vi "AT901 - Queue Steuerung.vi"() -> ()   [LabVIEW 2017]
uses:
  AT901 API/Structures/Struct SystemUnits.ctl
  AT901 API/TypeDefinitions/ES_LengthUnit.ctl
  AT901 API/TypeDefinitions/ES_AngleUnit.ctl
  AT901 API/TypeDefinitions/ES_TemperatureUnit.ctl
  AT901 API/TypeDefinitions/ES_PressureUnit.ctl
  AT901 API/TypeDefinitions/ES_HumidityUnit.ctl
  AT901 API/TypeDefinitions/ES_CoordinateSystemType.ctl
  AT901 API/Structures/Struct EnvironmentData.ctl
  AT901 API/Structures/Struct StationaryModeData.ctl
  AT901 API/TypeDefinitions/ES_ReflectorType.ctl
  AT901 API/Structures/Struct TransformationPoint.ctl
  TypeDefinitions/Queue Steuerung Commands.ctl
  AT901 API/TypeDefinitions/ES_MeasMode.ctl
  AT901 API/Structures/Struct ContinuousTimeModeData.ctl
  AT901 API/TypeDefinitions/ES_RegionType.ctl
  AT901 API/Structures/Struct SystemSettingsData.ctl
  AT901 API/TypeDefinitions/ES_WeatherMonitorStatus.ctl
  AT901 API/Structures/Struct TransformationData.ctl
  <vilib>/Analysis/baseanly.llb/Mean (DBL).vi
  <vilib>/Analysis/NI_AALBase.lvlib
panel:
  in  "Tab Control":T1(tab)
  in  "Connect":bool
  in  "Apply Transformation\nParameters":bool
  in  "Initialize":bool
  in  "GoBirdBath":bool
  in  "GetEnvParams":bool
  out "Environmental Data":T2
  in  "ContMeas":bool
  out "ContMeasResult":dbl[](array[numeric])
  out "Elements in Queue":i32
  in  "SingleMeas":bool
  out "SingleMeasResult":dbl[](array[numeric])
  in  "Punktnummer":string
  in  "Measurement File":path=path "C:/Users/Wehner/Desktop/AT901-MeasFile.txt"
  in  "IP Address":string="192.168.0.1"
  in  "Port":u16=700
  out "XY Graph":cluster{"Array":dbl[], "Array 3":dbl[]}(graph)
  in  "Axis Scaling":dbl(slide) scale=0.0..100.0
  in  "ES ReflectorType":T3=enum."CCR - 1,5 in"
  in  "ES_CoordinateSystemType":T4
  in  "SystemUnits":T5
  in  "Continuous Time Mode Params":T11={"TimeSeparation"=100, "NumberOfPoints"=0}
  in  "StationaryModeData":T12={"Use ADM"=TRUE, "lMeasTime"=500}
  in  "SetPowerLock\nActive":bool=TRUE
  out "Scale":dbl
  in  "Add Actual File":bool
  in  "Add Nominal File":bool
  out "Actual Points Front Indicator":T13(array[cluster])
  in  "Add Actual Point":bool
  in  "Clear Actual":bool
  in  "Remove Actual by Name":bool
  in  "Actual to be Removed":string
  out "Nominal Points Front Indicator":T13(array[cluster])
  in  "Clear Nominal":bool
  in  "Add Nominal":bool
  in  "Remove Nominal by Name":bool
  in  "Nominal to be Removes":string
  in  "CalcTransformation":bool
  out "Translation":dbl[](array[numeric])
  out "Rotation":dbl[](array[numeric])
  out "Nominal Points":T15(array[cluster])
  out "Actual Points":T15(array[cluster])
  # "Single Measurement"
  # "Continuous Measurement"
  # "General Settings"
  # "Continuous Measurement\nSettings"
  # "Single Measurement\nSettings"
  # "Set Nominal Points"
  # "Set Actual Points"
  # "Perform Transformation"
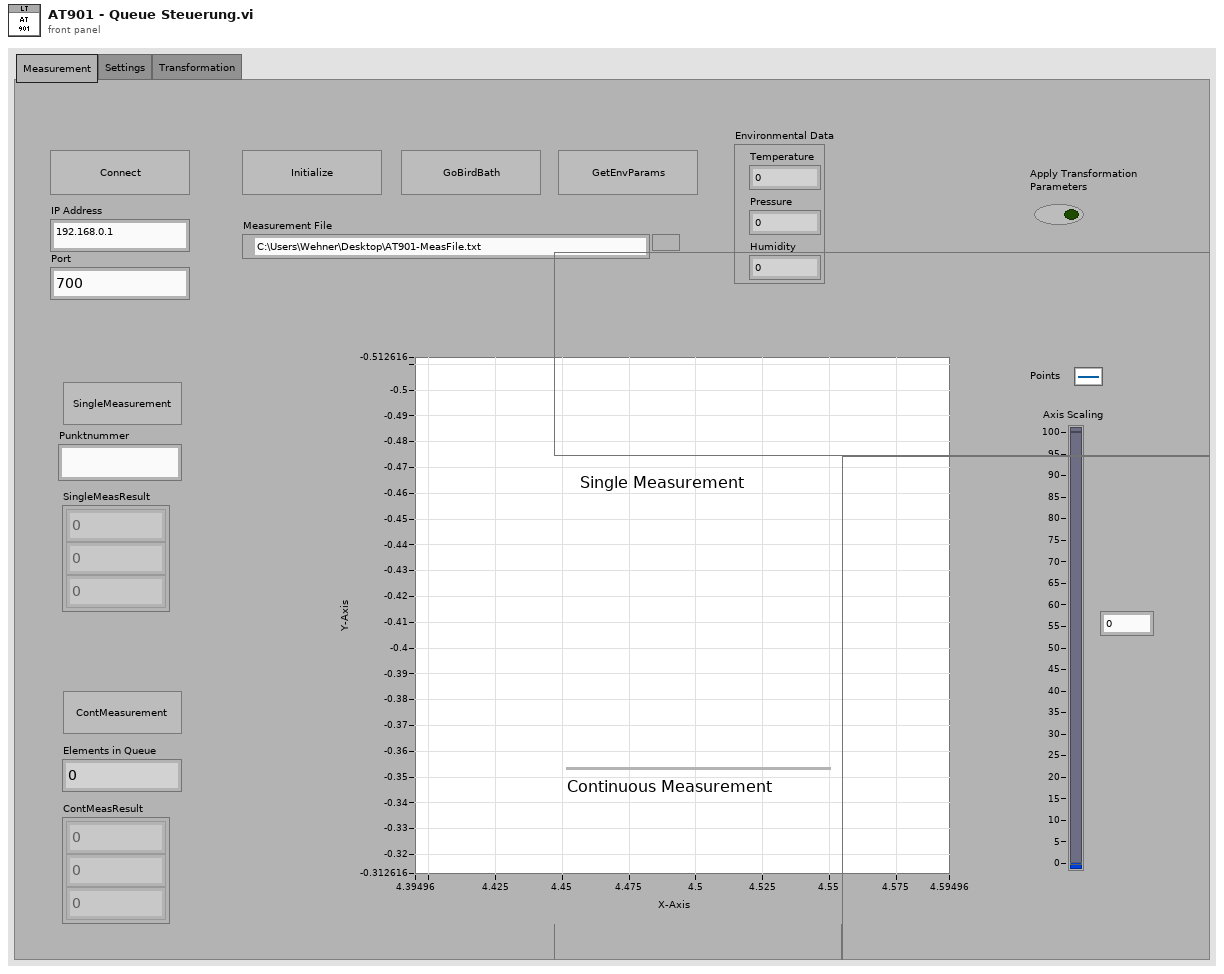
[diagram p1: front panel]
types:
  T1 = enum32{"Measurement", "Settings", "Transformation"}
  T2 = typedef "Struct EnvironmentData.ctl" = cluster{"Temperature":dbl, "Pressure":dbl, "Humidity":dbl}
  T3 = typedef "ES_ReflectorType.ctl" = enum32{"none1", "none2", "CCR - 1,5 in", "none4", "none5", "TBR - 0,5 in", "none7", "CCR - 75mm", "none8", "RRR - 1,5 in"}
  T4 = typedef "ES_CoordinateSystemType.ctl" = enum32{"ES_CS_RHR", "ES_CS_LHRX", "ES_CS_LHRY", "ES_CS_LHRZ", "ES_CS_CCW", "ES_CS_CCC", "ES_CS_SCW", "ES_CS_SCC"}
  T5 = typedef "Struct SystemUnits.ctl" = cluster{"ES_LengthUnit":T6, "ES_AngleUnit":T7, "ES_TemperatureUnit":T8, "ES_PressureUnit":T9, "ES_HumidityUnit":T10}
  T6 = typedef "ES_LengthUnit.ctl" = enum32{"ES_LU__Meter", "ES_LU_Millimeter", "ES_LU_Micron", "ES_LU_Foot", "ES_LU_Yard", "ES_LU_Inch"}
  T7 = typedef "ES_AngleUnit.ctl" = enum32{"ES_AU_Radian", "ES_AU_Degree", "ES_AU_Gon"}
  T8 = typedef "ES_TemperatureUnit.ctl" = enum32{"ES_TU_Celsius", "ES_TU_Fahrenheit"}
  T9 = typedef "ES_PressureUnit.ctl" = enum32{"ES_PU_Mbar", "ES_PU_HPascal", "ES_PU_KPascal", "ES_PU_MmHg", "ES_PU_Psi", "ES_PU_InH2O", "ES_PU_InHg"}
  T10 = typedef "ES_HumidityUnit.ctl" = enum32{"ES_HU_RH"}
  T11 = cluster{"TimeSeparation":u32, "NumberOfPoints":u32}
  T12 = typedef "Struct StationaryModeData.ctl" = cluster{"Use ADM":bool, "lMeasTime":i32}
  T13 = cluster{"X":dbl, "Y":dbl, "Z":dbl, "Punktnummer":string}[]
  T14 = typedef "Struct TransformationPoint.ctl" = cluster{"dVal1":dbl, "dVal2":dbl, "dVal3":dbl, "dStd1":dbl, "dStd2":dbl, "dStd3":dbl, "dCovar12":dbl, "dCovar13":dbl, "dCovar23":dbl}
  T15 = cluster{"Punktnummer":string, "Transformation Point":T14}[]
  T16 = typedef "Queue Steuerung Commands.ctl" = enum16{"Punkte Transformieren", "SetCoordType", "SetStatMeasParams", "AddNominalPoint", "ClearLastActualPoint", "ClearLastNominalPoint", "PowerLock", "AddActualPoint", "CalcTransformation", "SetContTimeParams", "GetEnvParams", "StopContMeas", "GetContMeasData", "StartContMeas", "Idle", "PlotValueChange", "ConnectTracker", "AddNominalPointFile", "AddActualPointFile", "RemoveNominalByName", "RemoveActualByName", "Stop", "Initialise", "SetUnits", "SetReflector", "SingleMeasurement", "GoBirdBath"}
  T17 = typedef "ES_MeasMode.ctl" = enum32{"ES_MM_Stationary", "ES_MM_ContinuousTime", "ES_MM_ContinuousDistance", "ES_MM_Grid", "ES_MM_SphrereCenter", "ES_MM_CircleCenter", "ES_MM_6DStationary", "ES_MM_6DContinuousTime", "ES_MM_6DContinuousDistance", "ES_MM_6DGrid", "ES_MM_6DSphrereCenter", "ES_MM6DCircleCenter"}
  T18 = typedef "Struct ContinuousTimeModeData.ctl" = cluster{"TimeSeparation":u32, "NumberOfPoints":u32, "UseRegion":bool, "ES_RegionType":T19}
  T19 = typedef "ES_RegionType.ctl" = enum32{"ES_RT_Sphere", "ES_RT_Box"}
  T20 = typedef "Struct SystemSettingsData.ctl" = cluster{"WeatherMonitorStatus":T21, "ApplyTransformationParams":bool, "ApplyStationOrientationParams":bool, "KeepLastPosition":bool, "SendUnsolicitedMessages":bool, "SendReflectorPositionData":bool, "TryMeasurementMode":bool, "HasNivel":bool, "HasVideoCamera":bool}
  T21 = typedef "ES_WeatherMonitorStatus.ctl" = enum16{"ES_WMS_NotConnected", "ES_WMS_ReadOnly", "ES_WMS_ReadAndCalculateRefractions"}
  T22 = typedef "Struct TransformationData.ctl" = cluster{"dVal1":dbl, "dVal2":dbl, "dVal3":dbl, "dRot1":dbl, "dRot2":dbl, "dRot3":dbl, "dScale":dbl}
  T23 = typedef "Struct TransformationPointWithPointnumber.ctl" = cluster{"Punktnummer":string, "Transformation Point":T14}
  T24 = typedef "Struct CallTrafo.ctl" = cluster{"dTransVal1":dbl, "dTransVal2":dbl, "dTransVal3":dbl, "dRot1":dbl, "dRot2":dbl, "dRot3":dbl, "dScale":dbl, "dTransVal1 Std":dbl, "dTransVal2 Std":dbl, "dTransVal3 Std":dbl, "dRot1 Std":dbl, "dRot2 Std":dbl, "dRot3 Std":dbl, "dScale Std":dbl, "dRMS":dbl, "dMaxDev":dbl, "dVarianceFactor":dbl}
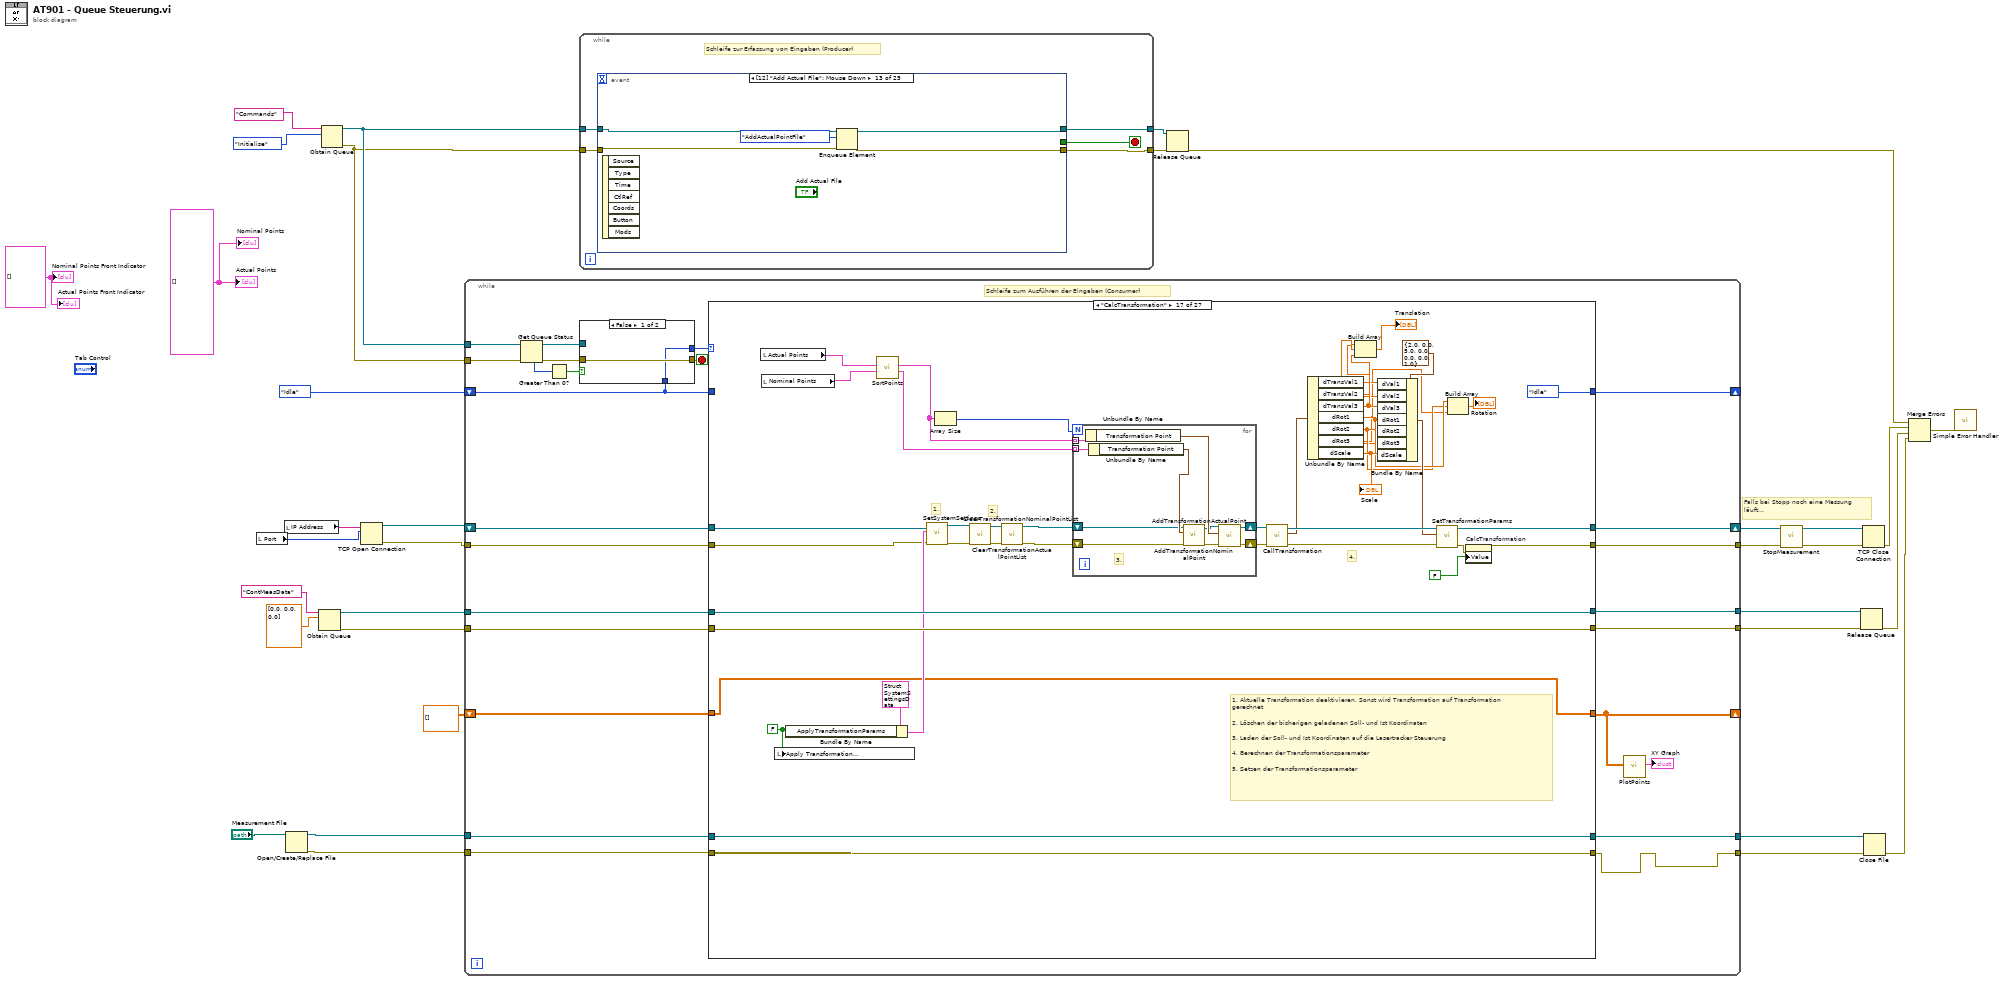
[diagram p0: block diagram]
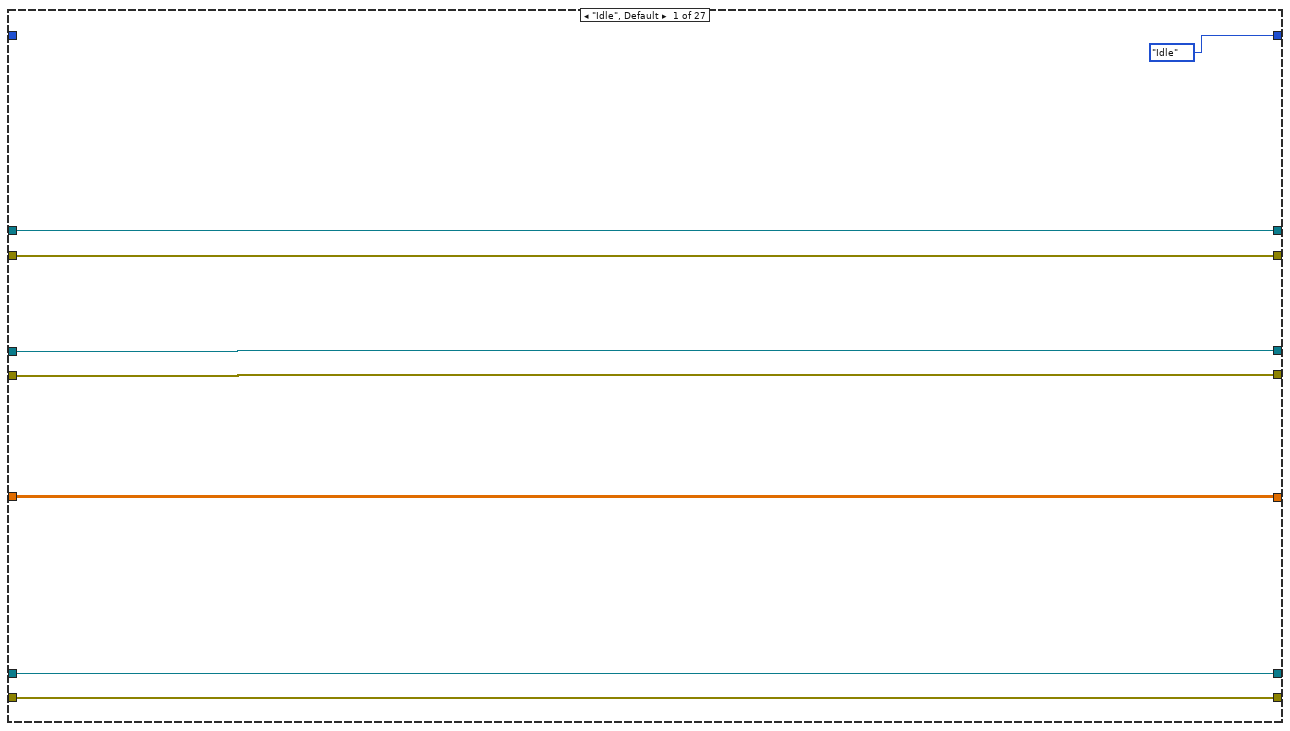
[diagram p2: hidden frame]
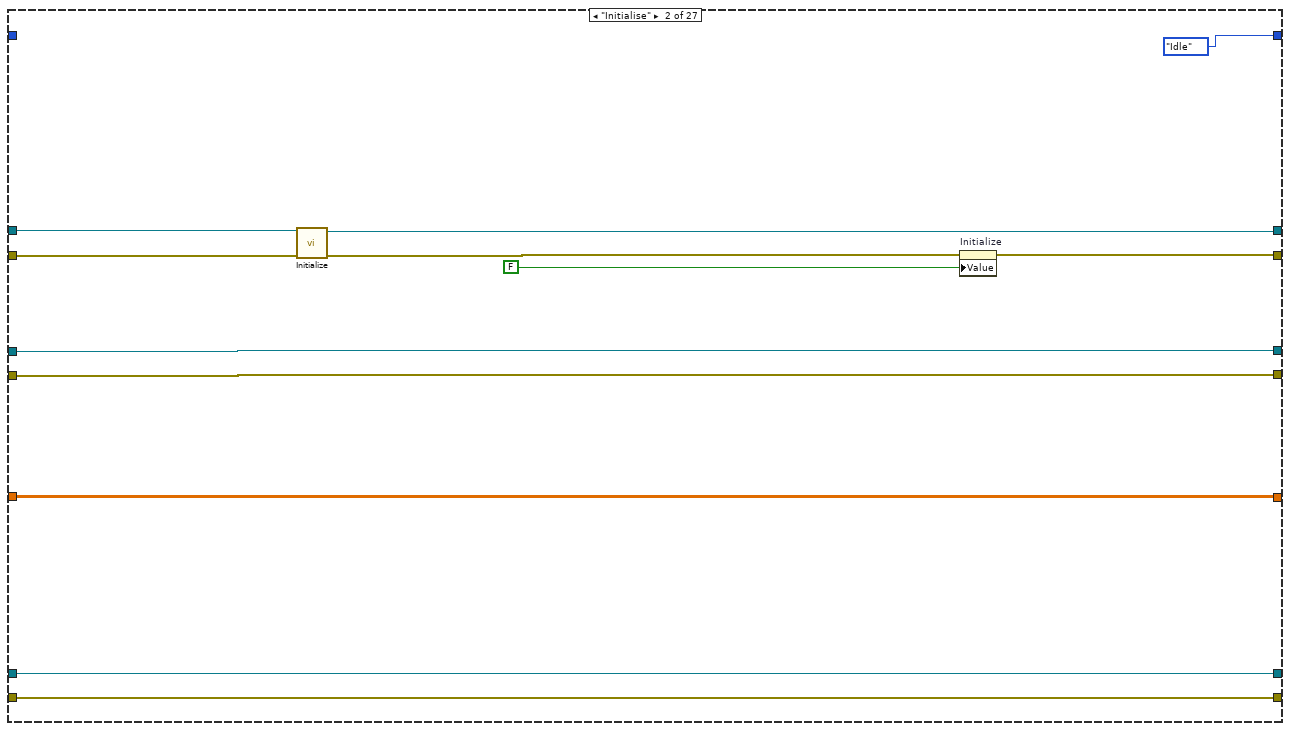
[diagram p3: hidden frame]
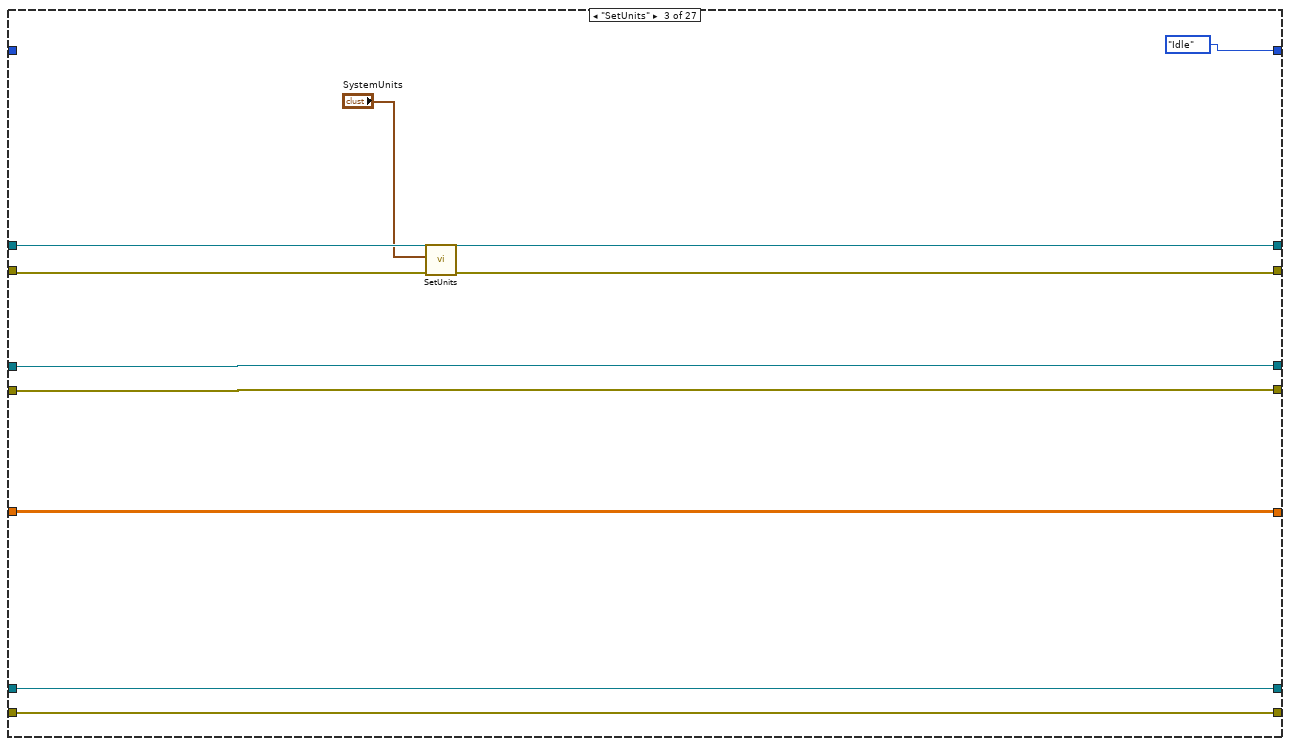
[diagram p4: hidden frame]
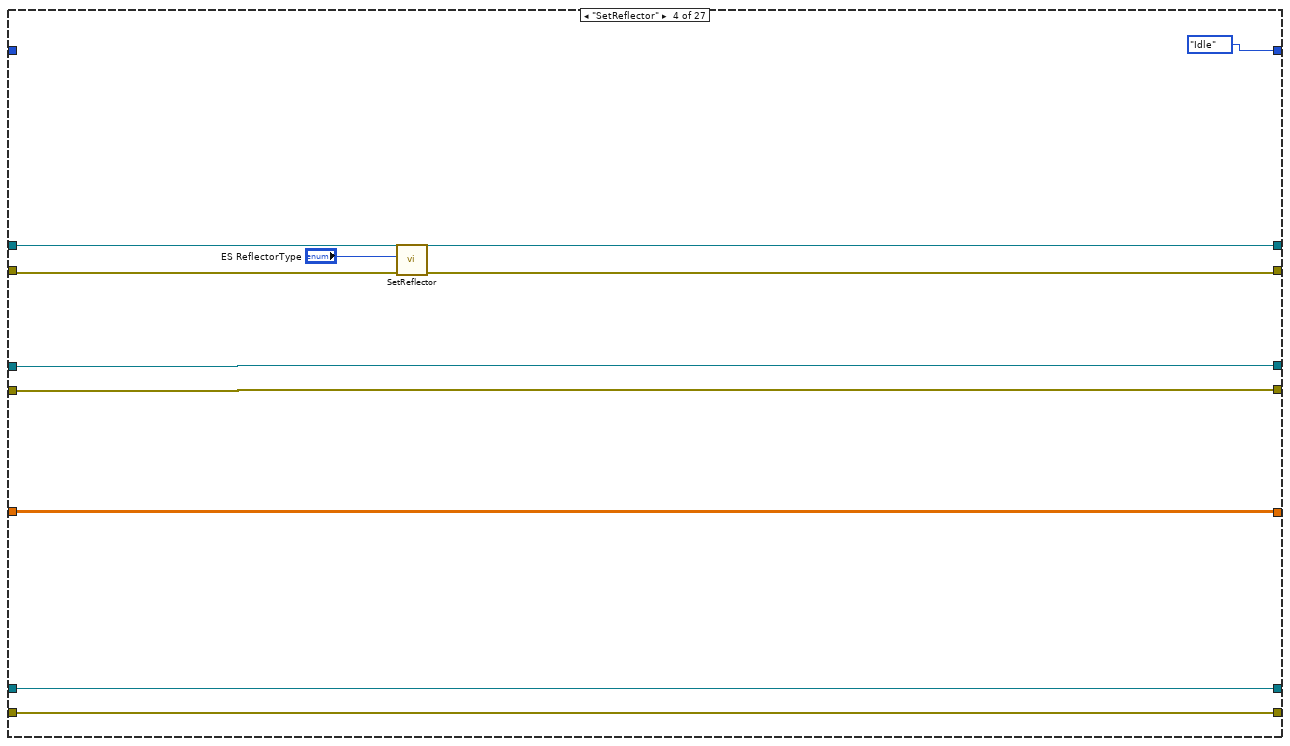
[diagram p5: hidden frame]
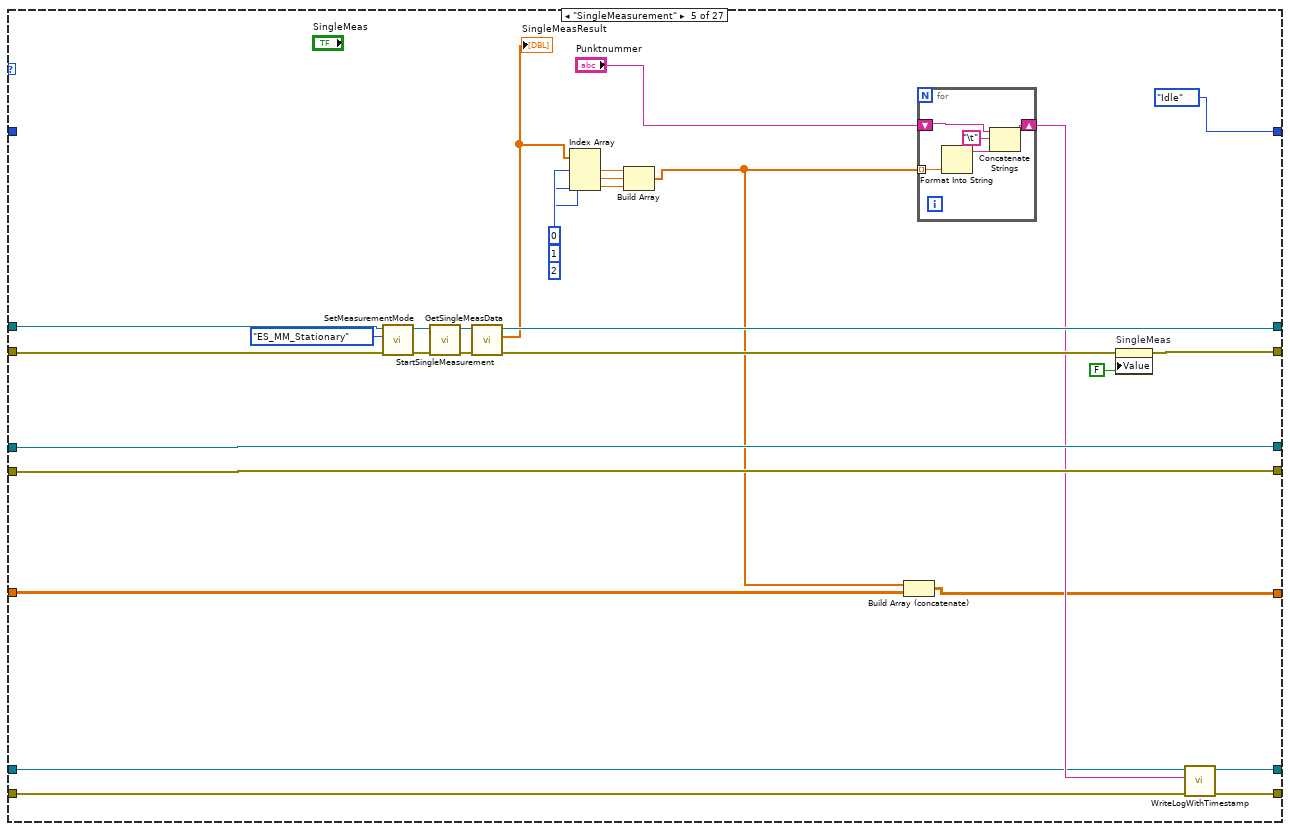
[diagram p6: hidden frame]
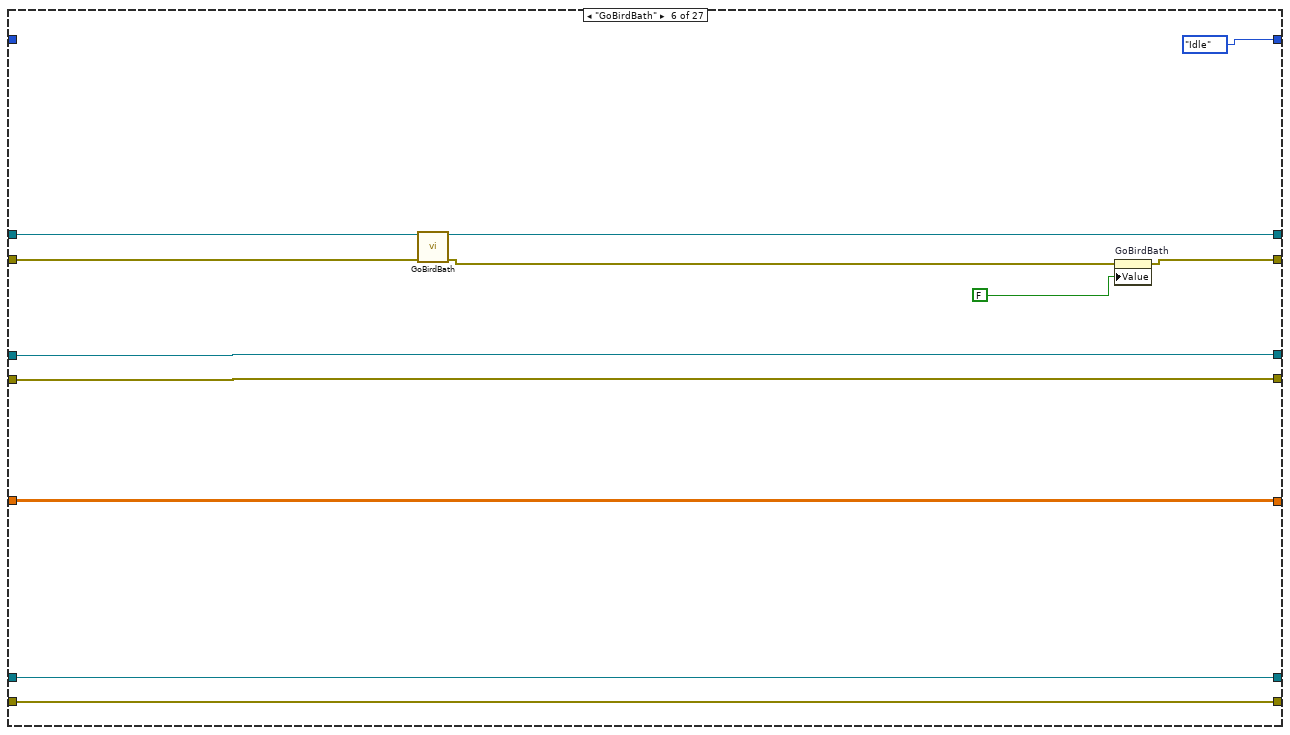
[diagram p7: hidden frame]
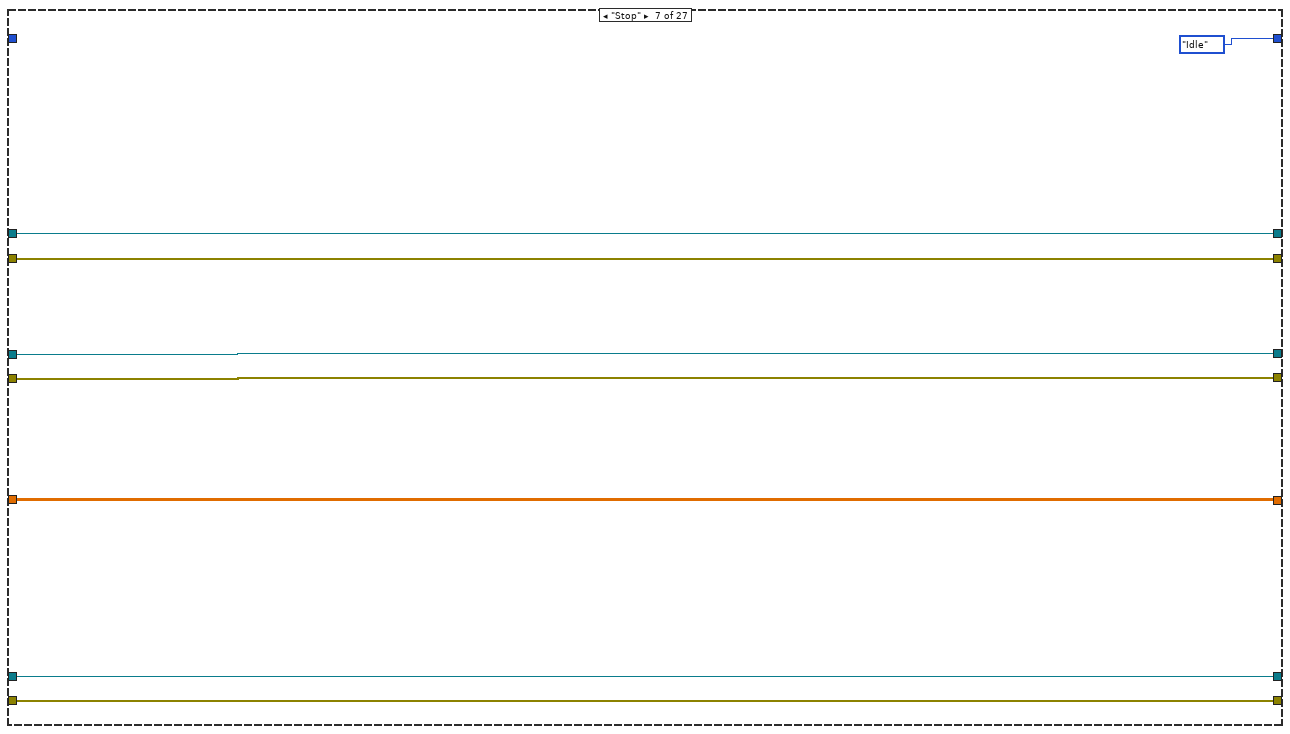
[diagram p8: hidden frame]
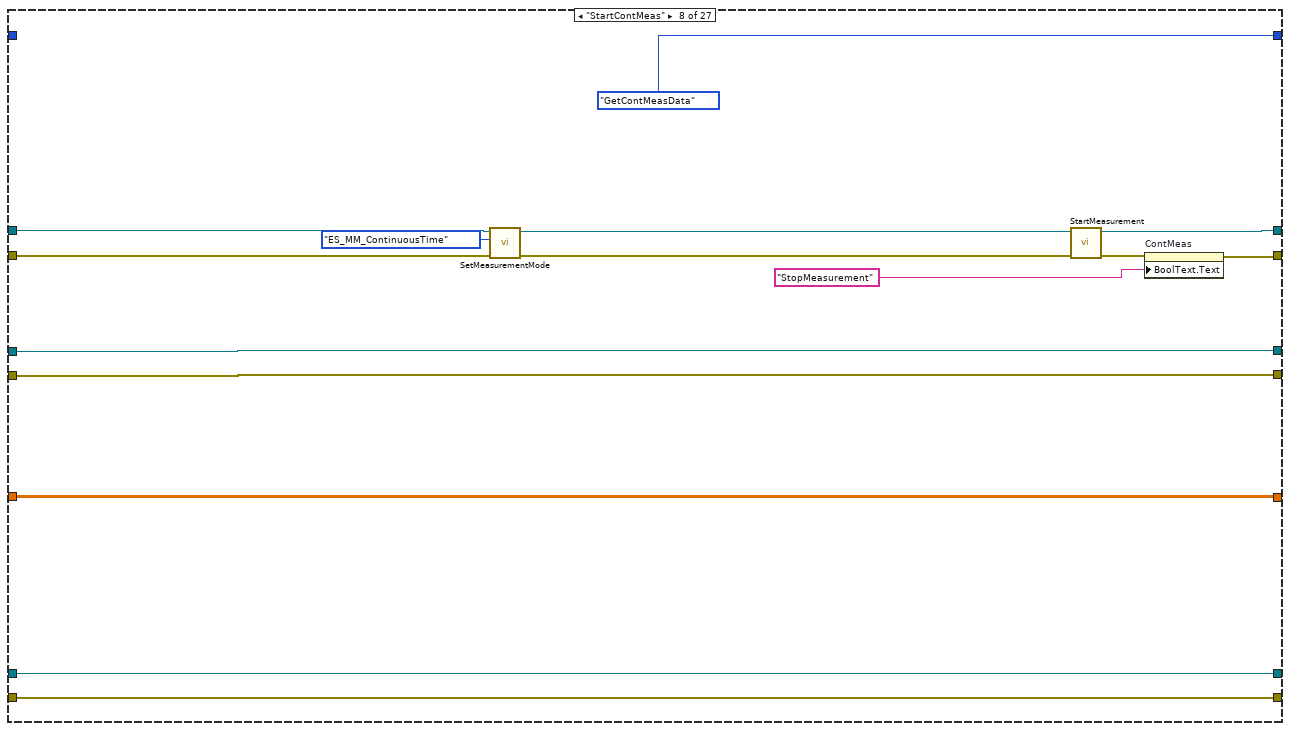
[diagram p9: hidden frame]
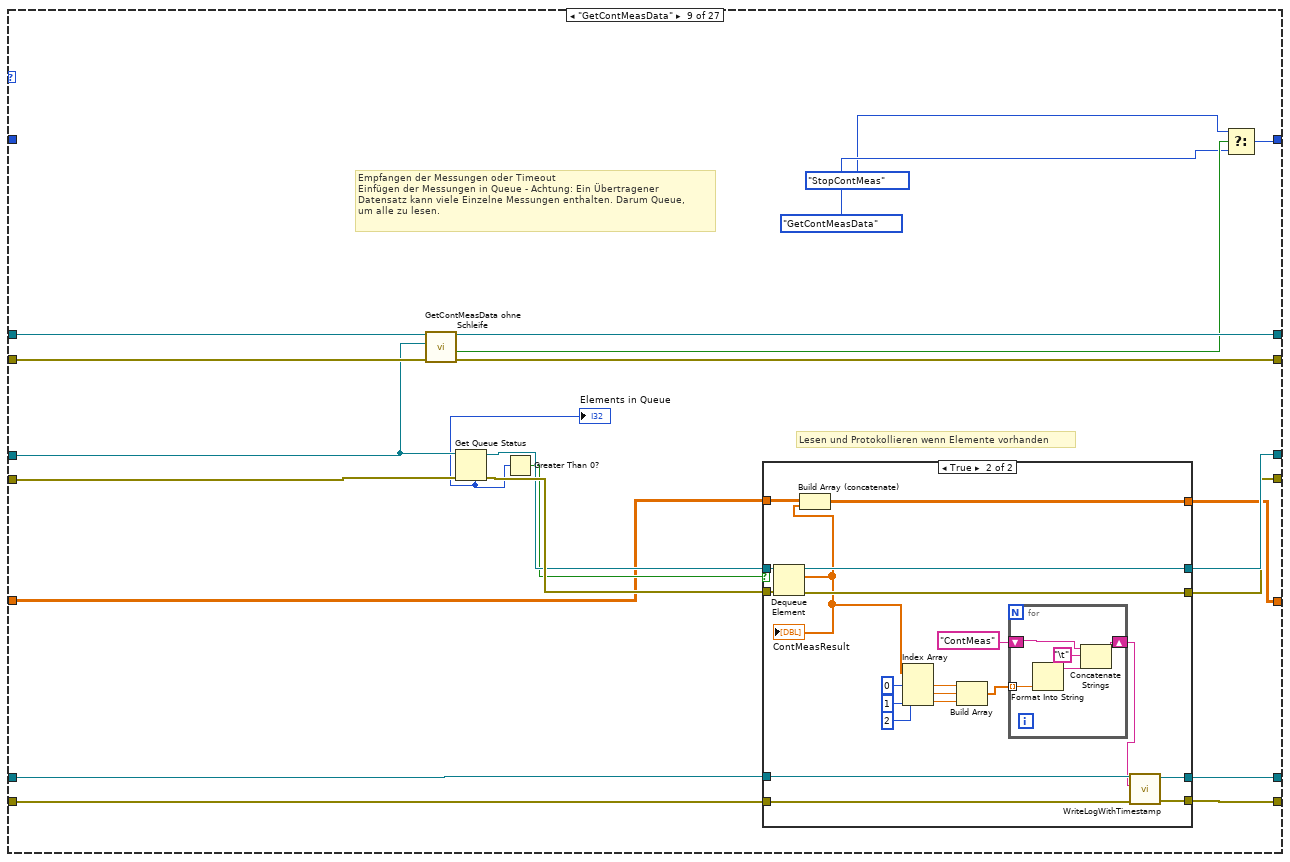
[diagram p10: hidden frame]
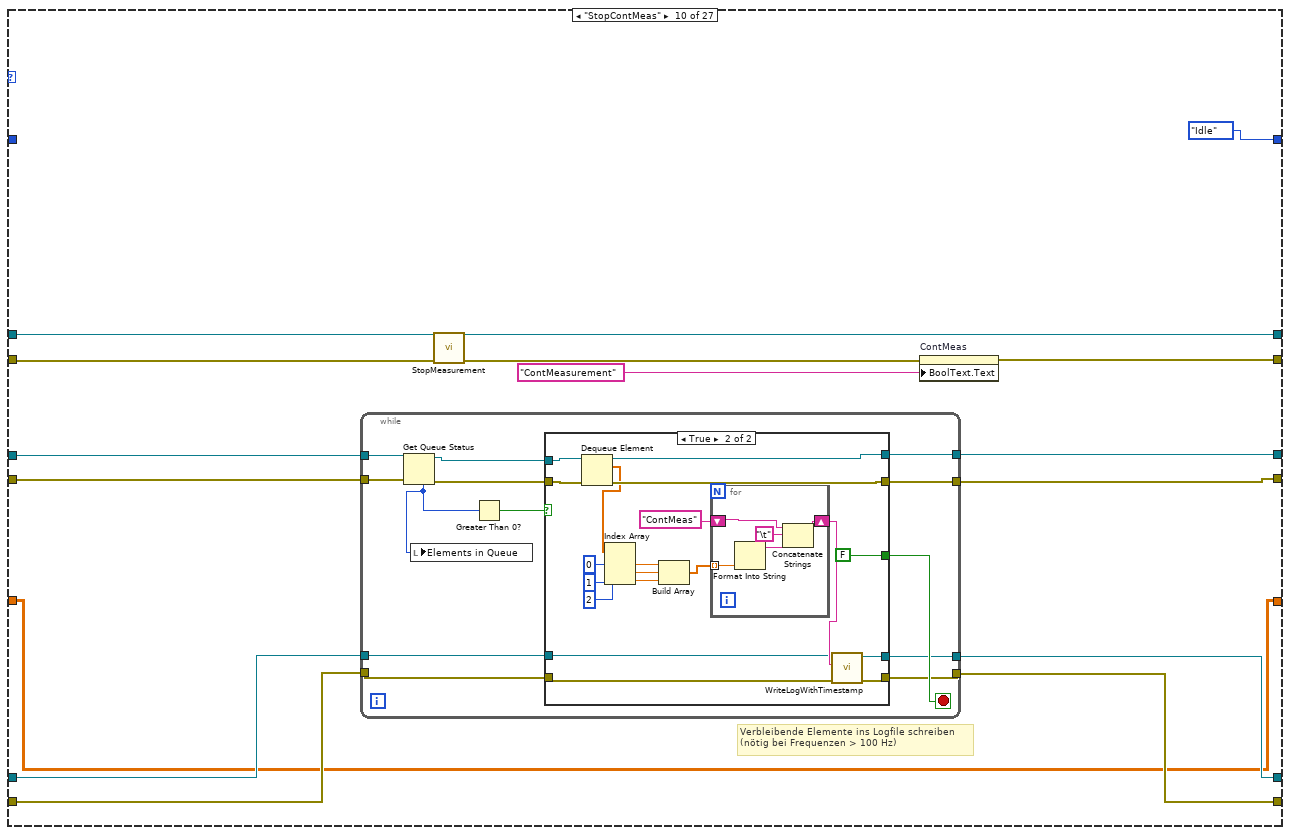
[diagram p12: hidden frame]
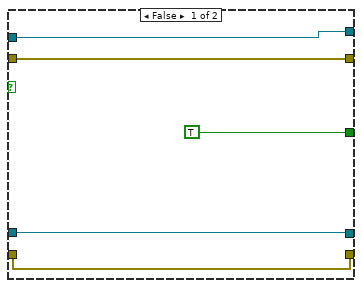
[diagram p13: hidden frame]
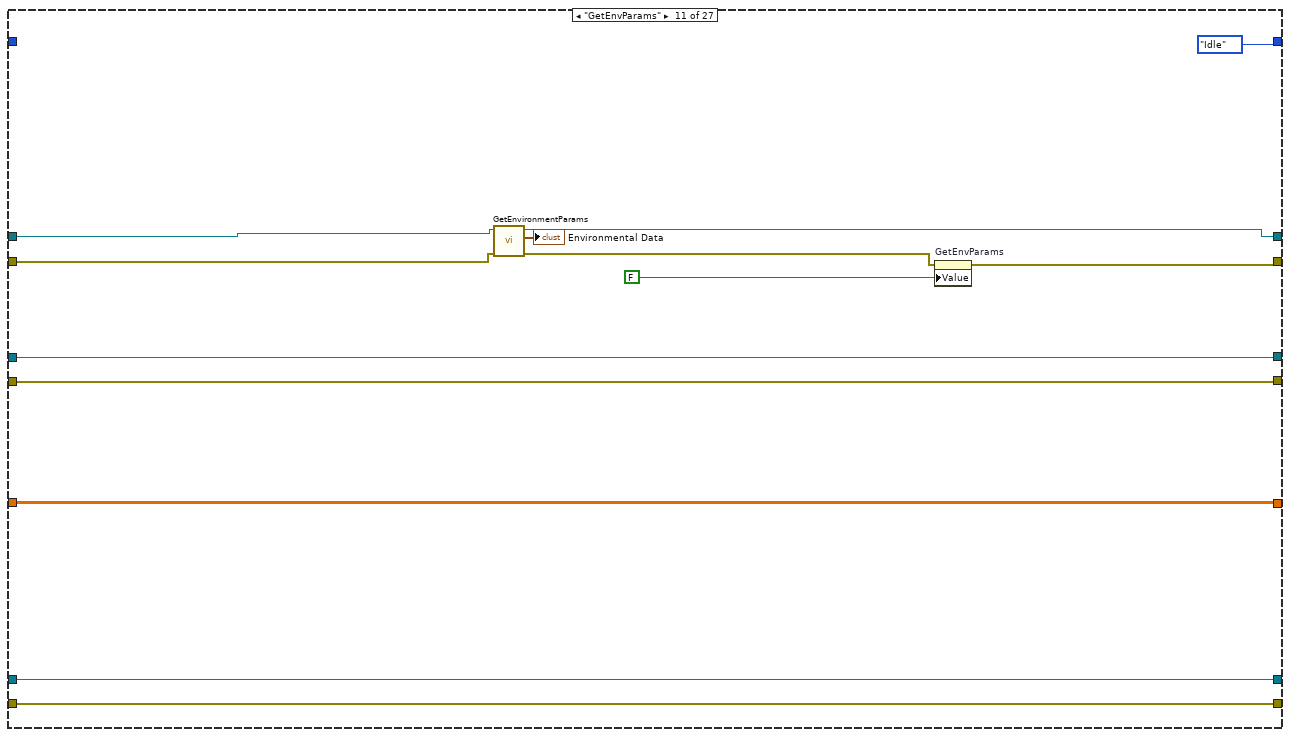
[diagram p14: hidden frame]
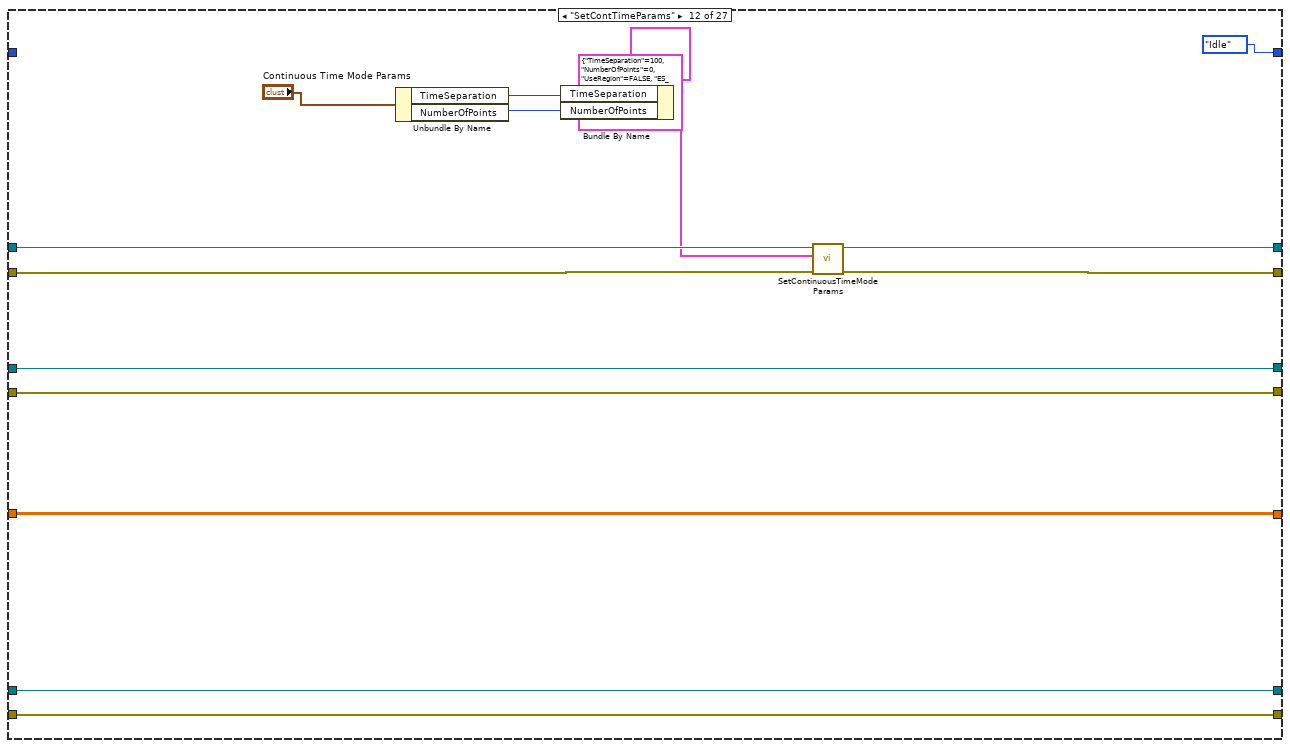
[diagram p15: hidden frame]
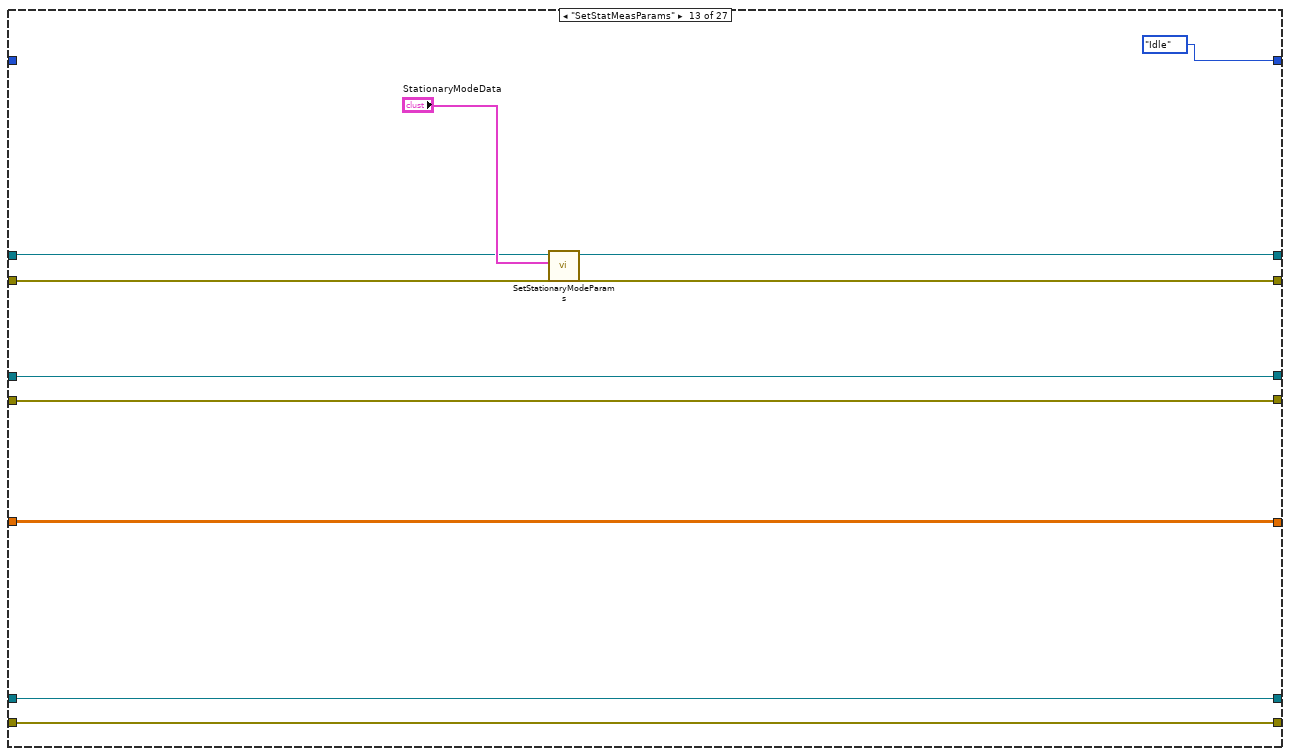
[diagram p16: hidden frame]
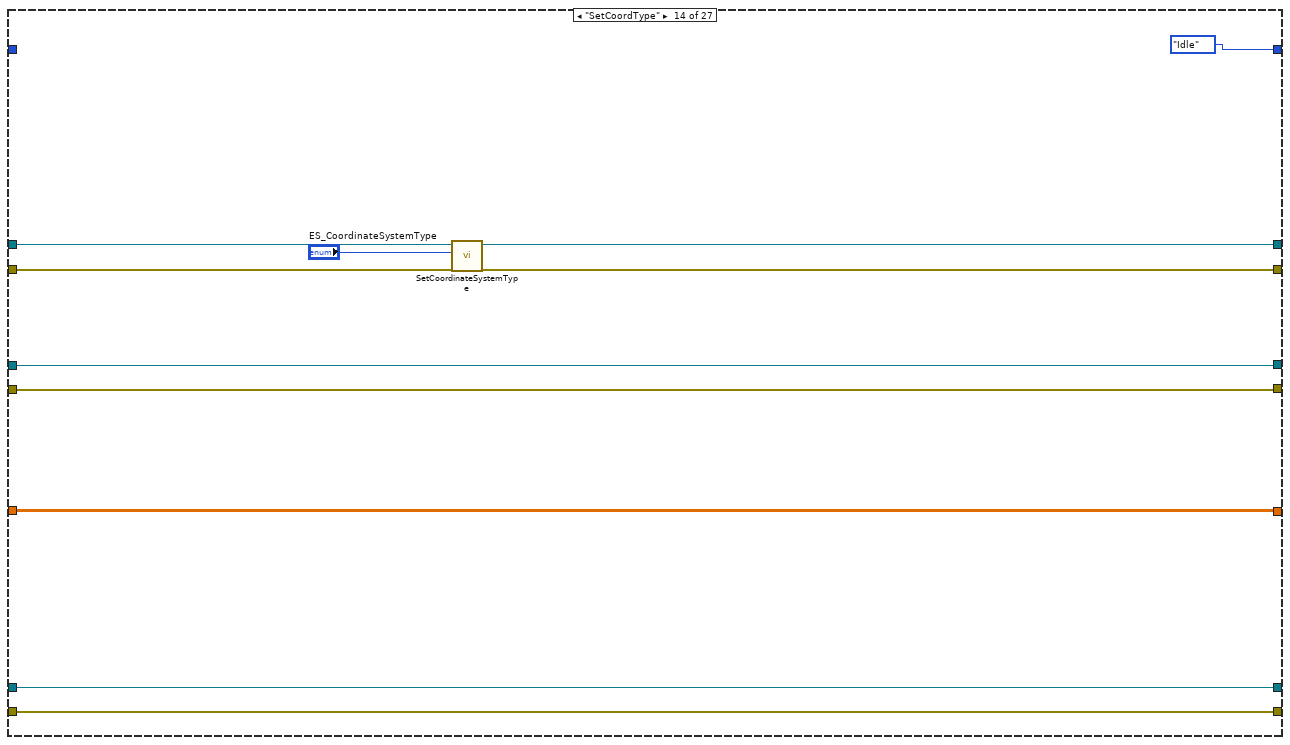
[diagram p17: hidden frame]
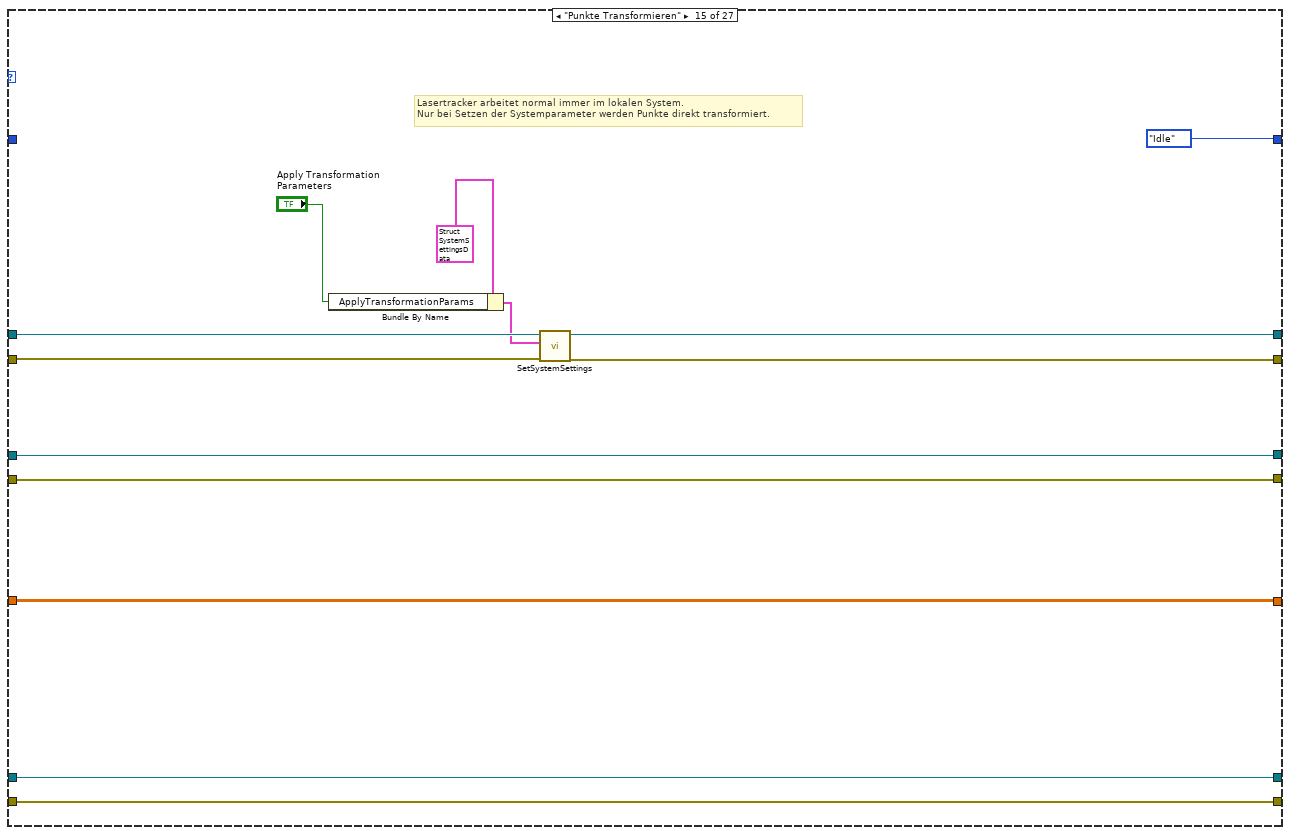
[diagram p18: hidden frame]
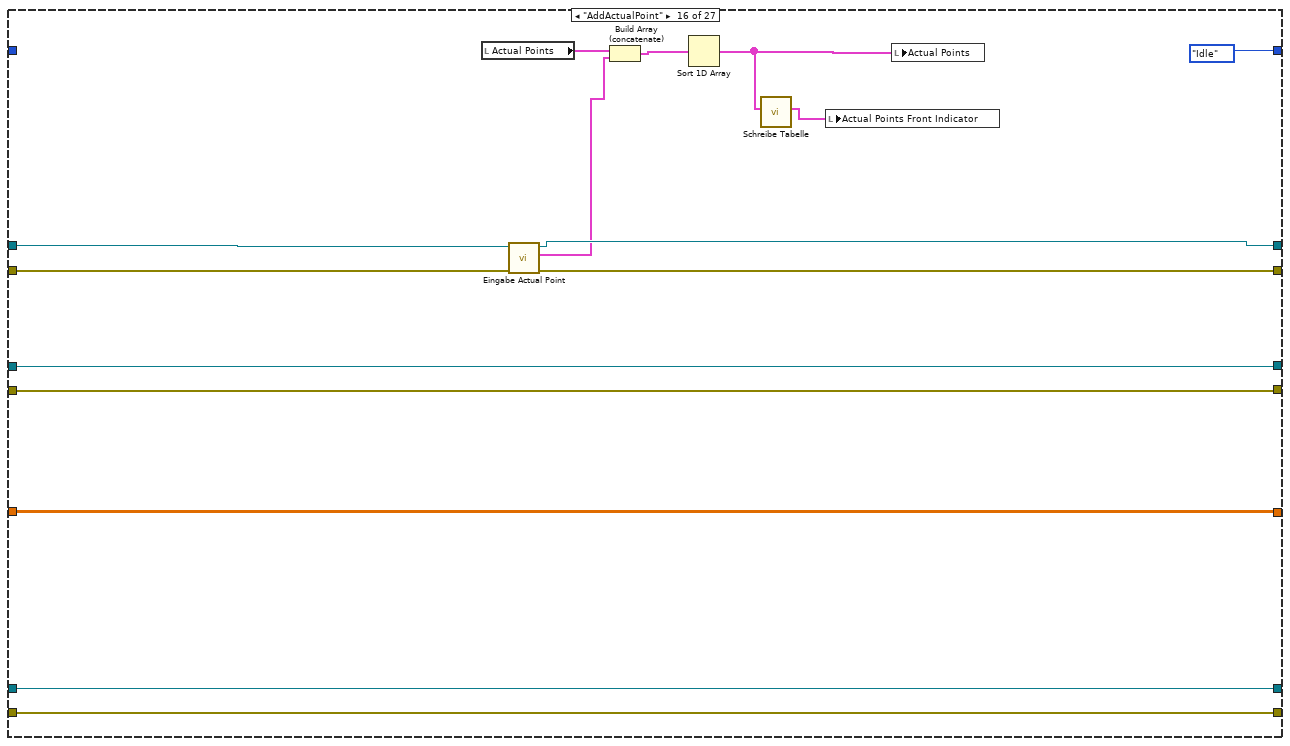
[diagram p19: hidden frame]
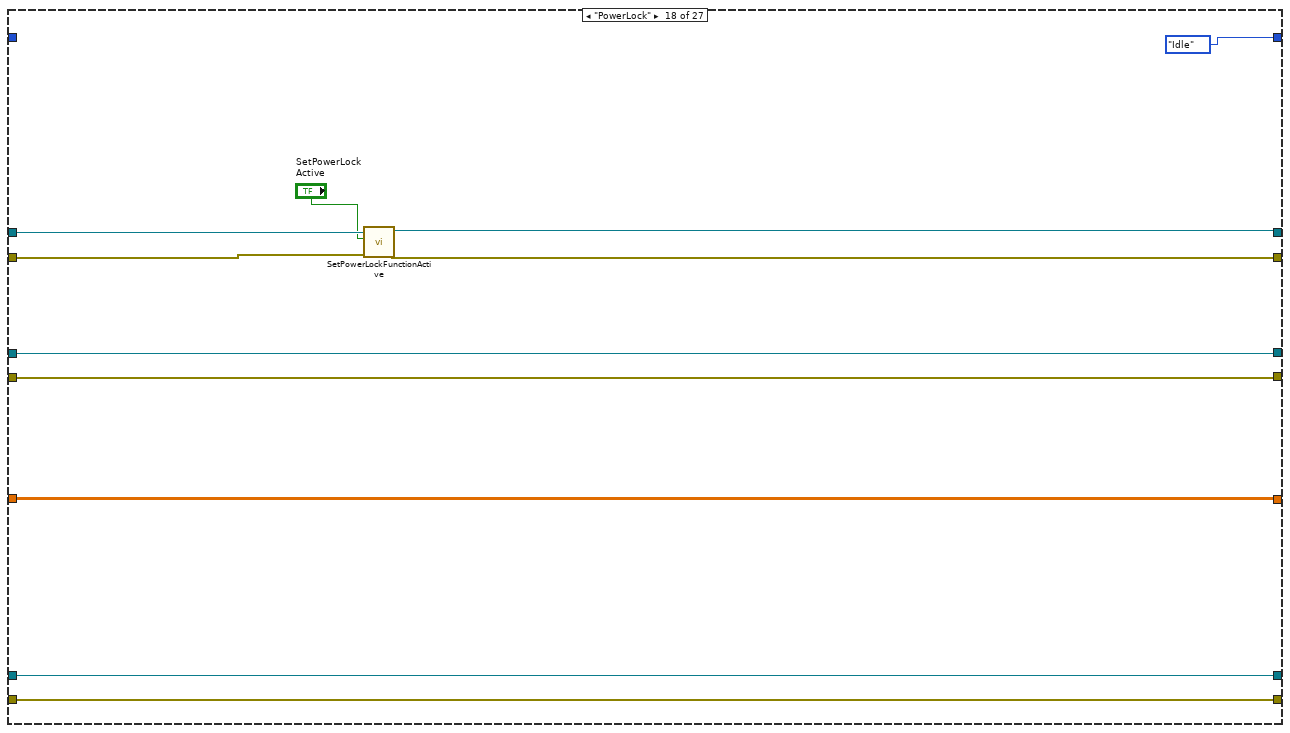
[diagram p20: hidden frame]
diagram:
  w13 = T13 [] ("Nominal Points")
  w14 = T15 [] ("Actual Points")
  # "Falls bei Stopp noch eine Messung\nläuft..."
  n1 = local read "Port"() -> (w4:u16)
  n2 = local read "IP Address"() -> (w5:string)
  n3 = Open/Create/Replace File(file path (use dialog)="Measurement File") -> (refnum out=w18:refnum<file>, error out=w2:errorcluster)  [unwired: 5 in, 1 out]
  n4 = Obtain Queue(name (unnamed)="ContMeasData", element data type=dbl[] [0.0, 0.0, 0.0] ("Meas Result")) -> (queue out=w25:refnum<queue>, error out=w24:errorcluster)  [unwired: 3 in, 1 out]
  n5 = Obtain Queue(name (unnamed)="Commands", element data type=Queue_Steuerung_Commands."Initialise") -> (queue out=w30:refnum<queue>, error out=w29:errorcluster)  [unwired: 3 in, 1 out]
  n6 = TCP Open Connection(address=w5, remote port or service name=w4) -> (connection ID=w7:refnum<k5>, error out=w6:errorcluster)  [unwired: 3 in]
  n7 = while {
    tunnel: w30 -> [w59]
    tunnel: w6 -> [w51]
    tunnel: [w50] -> w11
    tunnel: w29 -> [w49]
    shift-right: [w47] -> _
    shift-left: Queue_Steuerung_Commands."Idle" -> [w35]
    tunnel: w25 -> [w46]
    tunnel: w24 -> [w45]
    tunnel: [w44] -> w23
    tunnel: [w43] -> w22
    tunnel: w18 -> [w40]
    tunnel: w2 -> [w41]
    tunnel: [w42] -> w17
    shift-right: [w53] -> w8
    shift-left: w7 -> [w52]
    shift-right: [w38] -> _
    shift-left: dbl[][] [] -> [w39]
    tunnel: [w36] -> w1
    stop <- w48 stop-if-true
    # "Schleife zum Ausführen der Eingaben (Consumer)"
    n8 = Get Queue Status(queue=w59, error in (no error)=w49) -> (queue out=w57:refnum<queue>, error out=w56:errorcluster, # elements in queue=w58:i32)  [unwired: 1 in, 5 out]
    n9 = Greater Than 0?(x=w58) -> (x > 0?=w55:bool)
    n10 = case shown="False" w55 {
      tunnel: w57 -> [_ w558]
      tunnel: w56 -> [w554 w557]
      tunnel: [w553 w556] -> w54
      tunnel: [w554 w555] -> w48
      tunnel: w35 -> [w553 _]
      frame False {
      }
      frame True {
        n11 = Dequeue Element(queue=w558, error in (no error)=w557) -> (element=w556:T16, error out=w555:errorcluster)  [unwired: 1 in, 2 out]
      }
    }
    n12 = case shown="\"CalcTransformation\"" w54 {
      tunnel: [w67 w77 w85 w96 w126 w143 w156 w166 w190 w237 w290 w305 w315 w326 w338 w354 w391 w415 w435 w449 w463 w477 w491 w505 w519 w526 w552] -> w53
      tunnel: w52 -> [w67 w79 w88 w99 w129 w148 w156 w168 w193 w239 w292 w306 w317 w329 w340 w355 w382 w418 w435 w449 w463 w477 w491 w505 w519 _ w552]
      tunnel: w51 -> [w66 w78 w87 w98 w125 w147 w155 w167 w192 w238 w291 w307 w316 w328 w339 w352 w383 w417 w434 w448 w462 w467 w481 w494 w511 w525 w547]
      tunnel: [w66 w75 w86 w97 w121 w144 w155 w161 w191 w235 w286 w304 w314 w327 w337 w353 w376 w414 w434 w448 w462 w466 w482 w493 w510 w522 w546] -> w50
      tunnel: [Queue_Steuerung_Commands."Idle" Queue_Steuerung_Commands."Idle" Queue_Steuerung_Commands."Idle" Queue_Steuerung_Commands."Idle" Queue_Steuerung_Commands."Idle" Queue_Steuerung_Commands."Idle" Queue_Steuerung_Commands."Idle" Queue_Steuerung_Commands."GetContMeasData" w186 Queue_Steuerung_Commands."Idle" Queue_Steuerung_Commands."Idle" Queue_Steuerung_Commands."Idle" Queue_Steuerung_Commands."Idle" Queue_Steuerung_Commands."Idle" Queue_Steuerung_Commands."Idle" Queue_Steuerung_Commands."Idle" Queue_Steuerung_Commands."Idle" Queue_Steuerung_Commands."Idle" Queue_Steuerung_Commands."Idle" Queue_Steuerung_Commands."Idle" Queue_Steuerung_Commands."Idle" Queue_Steuerung_Commands."Idle" Queue_Steuerung_Commands."Idle" Queue_Steuerung_Commands."Idle" Queue_Steuerung_Commands."Idle" Queue_Steuerung_Commands."Idle" w534] -> w47
      tunnel: w46 -> [w65 w73 w90 w101 w120 w142 w154 w164 w183 w233 w294 w309 w320 w331 w344 w359 w401 w422 w433 w447 w461 w476 w490 w504 w518 w532 w551]
      tunnel: w45 -> [w64 w72 w89 w100 w119 w141 w153 w163 w182 w232 w293 w308 w319 w330 w343 w358 w400 w421 w432 w446 w460 w475 w489 w503 w517 w531 w550]
      tunnel: [w65 w73 w90 w101 w120 w142 w154 w164 w181 w230 w294 w309 w320 w331 w344 w359 w401 w422 w433 w447 w461 w476 w490 w504 w518 w532 w551] -> w44
      tunnel: [w64 w72 w89 w100 w119 w141 w153 w163 w180 w231 w293 w308 w319 w330 w343 w358 w400 w421 w432 w446 w460 w475 w489 w503 w517 w531 w550] -> w43
      tunnel: w41 -> [w63 w71 w83 w94 w106 w140 w152 w159 w175 w228 w285 w303 w313 w324 w342 w357 w399 w420 w431 w445 w459 w474 w488 w502 w516 w530 w549]
      tunnel: w40 -> [w62 w70 w82 w93 w107 w139 w151 w158 w174 w229 w284 w302 w312 w323 w341 w356 w398 w419 w430 w444 w458 w473 w487 w501 w515 w529 w548]
      tunnel: [w63 w71 w83 w94 w118 w140 w152 w159 w176 w227 w285 w303 w313 w324 w342 w357 w399 w420 w431 w445 w459 w474 w488 w502 w516 w530 w549] -> w36
      tunnel: [w62 w70 w82 w93 w117 w139 w151 w158 w177 w226 w284 w302 w312 w323 w341 w356 w398 w419 w430 w444 w458 w473 w487 w501 w515 w529 w548] -> w42
      tunnel: [w60 w68 w80 w91 w103 w137 w149 w157 w172 w224 w282 w295 w310 w321 w332 w345 w369 w412 w423 w436 w450 w464 w478 w492 w506 w520 w544] -> w38
      tunnel: w39 -> [w60 w68 w80 w91 w102 w137 w149 w157 w173 w224 w282 w295 w310 w321 w332 w345 w369 w412 w423 w436 w450 w464 w478 w492 w506 w520 w544]
      tunnel: w35 -> [_ _ _ _ _ _ _ _ _ _ _ _ _ _ _ _ _ _ _ _ _ _ _ _ _ _ w534]
      frame "Idle", Default {
      }
      frame "Initialise" {
        n13 = call "Initialize.vi"("error in (no error)"=w78, "TCP Network Connection in"=w79) -> ("error out"=w76:errorcluster, "TCP Network Connection out"=w77:refnum<k5>)  [unwired: 6 in, 2 out]
        n14 = property on="Initialize" class="Bool (strict)"(error in=w76, "Value"=FALSE ("Initialize")) -> (error out=w75:errorcluster)  [unwired: 1 in, 1 out]
      }
      frame "SetUnits" {
        n15 = call "SetUnits.vi"("error in (no error)"=w87, "SystemUnits"="SystemUnits", "TCP Network Connection in"=w88) -> ("error out"=w86:errorcluster, "TCP Network Connection out"=w85:refnum<k5>)  [unwired: 5 in, 2 out]
      }
      frame "SetReflector" {
        n16 = call "SetReflector.vi"("error in (no error)"=w98, "ES ReflectorType"="ES ReflectorType", "TCP Network Connection in"=w99) -> ("error out"=w97:errorcluster, "TCP Network Connection out"=w96:refnum<k5>)  [unwired: 5 in, 2 out]
      }
      frame "SingleMeasurement" {
        n17 = call "SetMeasurementMode.vi"("error in (no error)"=w125, "ES_MeasMode"=ES_MeasMode."ES_MM_Stationary", "TCP Network Connection in"=w129) -> ("error out"=w130:errorcluster, "TCP Network Connection out"=w128:refnum<k5>)  [unwired: 5 in, 2 out]
        n18 = call "StartSingleMeasurement.vi"("error in (no error)"=w130, "TCP Network Connection in"=w128) -> ("error out"=w131:errorcluster, "TCP Network Connection out"=w127:refnum<k5>)  [unwired: 7 in, 1 out]
        n19 = call "GetSingleMeasData.vi"("error in (no error)"=w131, "TCP Network Connection in"=w127) -> ("error out"=w122:errorcluster, "Meas Result"=w113:dbl[], "TCP Network Connection out"=w126:refnum<k5>)  [unwired: 6 in, 1 out]
        "SingleMeasResult" <- w113
        n20 = Index Array(array=w113, index #1=0 ("index"), index #2=1 ("index"), index #3=2 ("index")) -> (element #1=w112:dbl, element #2=w111:dbl, element #3=w110:dbl)
        n21 = Build Array(w112, w111, w110) -> (w104:dbl[])
        n22 = Build Array (concatenate)(w104, w102) -> (w103:dbl[][])
        n23 = for {
          tunnel: w104 -> [w136] mode=indexing
          shift-right: [w133] -> w108
          shift-left: "Punktnummer" -> [w134]
          n24 = Format Into String(w136) -> (resulting string=w135:string)  [unwired: 3 in, 1 out]
          n25 = Concatenate Strings(w134, "\t", w135) -> (w133:string)
        }
        n26 = property on="SingleMeas" class="Bool (strict)"(error in=w122, "Value"=FALSE ("SingleMeas")) -> (error out=w121:errorcluster)  [unwired: 1 in, 1 out]
        n27 = call "WriteLogWithTimestamp.vi"("error in (no error)"=w106, "Punktnummer"=w108, "Byte Stream File in"=w107) -> ("error out"=w118:errorcluster, "Byte Stream File out"=w117:refnum<file>)  [unwired: 7 in]
      }
      frame "GoBirdBath" {
        n28 = call "GoBirdBath.vi"("error in (no error)"=w147, "TCP Network Connection in"=w148) -> ("error out"=w145:errorcluster, "TCP Network Connection out"=w143:refnum<k5>)  [unwired: 6 in, 2 out]
        n29 = property on="GoBirdBath" class="Bool (strict)"(error in=w145, "Value"=FALSE ("GoBirdBath")) -> (error out=w144:errorcluster)  [unwired: 1 in, 1 out]
      }
      frame "Stop" {
      }
      frame "StartContMeas" {
        n30 = call "SetMeasurementMode.vi"("error in (no error)"=w167, "ES_MeasMode"=ES_MeasMode."ES_MM_ContinuousTime", "TCP Network Connection in"=w168) -> ("error out"=w170:errorcluster, "TCP Network Connection out"=w169:refnum<k5>)  [unwired: 5 in, 2 out]
        n31 = call "StartMeasurement.vi"("error in (no error)"=w170, "TCP Network Connection in"=w169) -> ("error out"=w162:errorcluster, "TCP Network Connection out"=w166:refnum<k5>)  [unwired: 6 in, 2 out]
        n32 = property on="ContMeas" class="Bool (strict)"(error in=w162, "BoolText.Text"="StopMeasurement" ("Boolean Text.Text")) -> (error out=w161:errorcluster)  [unwired: 1 in, 1 out]
      }
      frame "GetContMeasData" {
        # "Lesen und Protokollieren wenn Elemente vorhanden"
        # "Empfangen der Messungen oder Timeout\nEinfügen der Messungen in Queue - Achtung: Ein Übertragener\nDatensatz kann viele Einzelne Messungen enthalten. Darum Queue, \num alle zu lesen."
        n33 = call "GetContMeasData ohne Schleife.vi"("error in (no error)"=w192, "queue out"=w183, "TCP Network Connection in"=w193) -> ("error out"=w191:errorcluster, "Messabbruch"=w189:bool, "TCP Network Connection out"=w190:refnum<k5>)  [unwired: 4 in, 2 out]
        n34 = Get Queue Status(queue=w183, error in (no error)=w182) -> (queue out=w184:refnum<queue>, error out=w185:errorcluster, # elements in queue=w178:i32)  [unwired: 1 in, 5 out]
        "Elements in Queue" <- w178
        n35 = Greater Than 0?(x=w178) -> (x > 0?=w179:bool)
        n36 = case shown="True" w179 {
          tunnel: w185 -> [w197 w218]
          tunnel: w184 -> [w198 w217]
          tunnel: [w198 w216] -> w181
          tunnel: [w197 w215] -> w180
          tunnel: [w196 w214] -> w177
          tunnel: [w195 w213] -> w176
          tunnel: w175 -> [w195 w212]
          tunnel: w174 -> [w196 w211]
          tunnel: w173 -> [w194 w201]
          tunnel: [w194 w199] -> w172
          frame False {
          }
          frame True {
            n37 = Dequeue Element(queue=w217, error in (no error)=w218) -> (queue out=w216:refnum<queue>, element=w200:dbl[], error out=w215:errorcluster)  [unwired: 1 in, 1 out]
            "ContMeasResult" <- w200
            n38 = Build Array (concatenate)(w201, w200) -> (w199:dbl[][])
            n39 = Index Array(array=w200, index #1=0 ("index"), index #2=1 ("index"), index #3=2 ("index")) -> (element #1=w207:dbl, element #2=w206:dbl, element #3=w205:dbl)
            n40 = Build Array(w207, w206, w205) -> (w204:dbl[])
            n41 = for {
              tunnel: w204 -> [w223] mode=indexing
              shift-right: [w220] -> w203
              shift-left: "ContMeas" -> [w221]
              n42 = Format Into String(w223) -> (resulting string=w222:string)  [unwired: 3 in, 1 out]
              n43 = Concatenate Strings(w221, "\t", w222) -> (w220:string)
            }
            n44 = call "WriteLogWithTimestamp.vi"("error in (no error)"=w212, "Punktnummer"=w203, "Byte Stream File in"=w211) -> ("error out"=w213:errorcluster, "Byte Stream File out"=w214:refnum<file>)  [unwired: 7 in]
          }
        }
        n45 = Select(t=Queue_Steuerung_Commands."StopContMeas", s=w189, f=Queue_Steuerung_Commands."GetContMeasData") -> (s? t:f=w186:T16)
      }
      frame "StopContMeas" {
        # "Verbleibende Elemente ins Logfile schreiben\n(nötig bei Frequenzen > 100 Hz)"
        n46 = while {
          tunnel: w233 -> [w252]
          tunnel: w232 -> [w251]
          tunnel: [w248] -> w231
          tunnel: [w245] -> w230
          tunnel: w229 -> [w244]
          tunnel: w228 -> [w243]
          tunnel: [w242] -> w227
          tunnel: [w241] -> w226
          stop <- w249 stop-if-true
          n47 = Get Queue Status(queue=w252, error in (no error)=w251) -> (queue out=w246:refnum<queue>, error out=w247:errorcluster, # elements in queue=w240:i32)  [unwired: 1 in, 5 out]
          n48 = local write "Elements in Queue"(w240) -> ()
          n49 = Greater Than 0?(x=w240) -> (x > 0?=w250:bool)
          n50 = case shown="True" w250 {
            tunnel: [TRUE FALSE] -> w249
            tunnel: [w256 w274] -> w248
            tunnel: w247 -> [w256 w272]
            tunnel: w246 -> [w255 w273]
            tunnel: [w255 w275] -> w245
            tunnel: w244 -> [w254 w262]
            tunnel: w243 -> [w253 w261]
            tunnel: [w253 w259] -> w242
            tunnel: [w254 w258] -> w241
            frame False {
            }
            frame True {
              n51 = Dequeue Element(queue=w273, error in (no error)=w272) -> (queue out=w275:refnum<queue>, element=w260:dbl[], error out=w274:errorcluster)  [unwired: 1 in, 1 out]
              n52 = Index Array(array=w260, index #1=0 ("index"), index #2=1 ("index"), index #3=2 ("index")) -> (element #1=w268:dbl, element #2=w267:dbl, element #3=w266:dbl)
              n53 = Build Array(w268, w267, w266) -> (w265:dbl[])
              n54 = for {
                tunnel: w265 -> [w281] mode=indexing
                shift-right: [w278] -> w264
                shift-left: "ContMeas" -> [w279]
                n55 = Format Into String(w281) -> (resulting string=w280:string)  [unwired: 3 in, 1 out]
                n56 = Concatenate Strings(w279, "\t", w280) -> (w278:string)
              }
              n57 = call "WriteLogWithTimestamp.vi"("error in (no error)"=w261, "Punktnummer"=w264, "Byte Stream File in"=w262) -> ("error out"=w259:errorcluster, "Byte Stream File out"=w258:refnum<file>)  [unwired: 7 in]
            }
          }
        }
        n58 = call "StopMeasurement.vi"("error in (no error)"=w238, "TCP Network Connection in"=w239) -> ("error out"=w236:errorcluster, "TCP Network Connection out"=w237:refnum<k5>)  [unwired: 6 in, 2 out]
        n59 = property on="ContMeas" class="Bool (strict)"(error in=w236, "BoolText.Text"="ContMeasurement" ("Boolean Text.Text")) -> (error out=w235:errorcluster)  [unwired: 1 in, 1 out]
      }
      frame "GetEnvParams" {
        n60 = call "GetEnvironmentParams.vi"("error in (no error)"=w291, "TCP Network Connection in"=w292) -> ("error out"=w287:errorcluster, "Environmental Data"=→"Environmental Data":T2, "TCP Network Connection out"=w290:refnum<k5>)  [unwired: 5 in, 2 out]
        n61 = property on="GetEnvParams" class="Bool (strict)"(error in=w287, "Value"=FALSE ("GetEnvParams")) -> (error out=w286:errorcluster)  [unwired: 1 in, 1 out]
      }
      frame "SetContTimeParams" {
        n62 = Unbundle By Name("Continuous Time Mode Params") -> ("TimeSeparation"=w298:u32, "NumberOfPoints"=w297:u32)
        n63 = Bundle By Name(cluster=T18 {"TimeSeparation"=100, "NumberOfPoints"=0, "UseRegion"=FALSE, "ES_RegionType"=enum."ES_RT_Sphere"} ("ContinuousTimeModeData"), "TimeSeparation"=w298, "NumberOfPoints"=w297) -> (w300:T18)
        n64 = call "SetContinuousTimeModeParams.vi"("error in (no error)"=w307, "ContinuousTimeModeData"=w300, "TCP Network Connection in"=w306) -> ("error out"=w304:errorcluster, "TCP Network Connection out"=w305:refnum<k5>)  [unwired: 5 in, 2 out]
      }
      frame "SetStatMeasParams" {
        n65 = call "SetStationaryModeParams.vi"("error in (no error)"=w316, "StationaryModeData"="StationaryModeData", "TCP Network Connection in"=w317) -> ("error out"=w314:errorcluster, "TCP Network Connection out"=w315:refnum<k5>)  [unwired: 5 in, 2 out]
      }
      frame "SetCoordType" {
        n66 = call "SetCoordinateSystemType.vi"("error in (no error)"=w328, "ES_CoordinateSystemType"="ES_CoordinateSystemType", "TCP Network Connection in"=w329) -> ("error out"=w327:errorcluster, "TCP Network Connection out"=w326:refnum<k5>)  [unwired: 5 in, 2 out]
      }
      frame "Punkte Transformieren" {
        # "Lasertracker arbeitet normal immer im lokalen System. \nNur bei Setzen der Systemparameter werden Punkte direkt transformiert."
        n67 = Bundle By Name(cluster=T20 {"WeatherMonitorStatus"=enum."ES_WMS_ReadAndCalculateRefractions", "ApplyTransformationParams"=FALSE, "ApplyStationOrientationParams"=FALSE, "KeepLastPosition"=TRUE, "SendUnsolicitedMessages"=TRUE, "SendReflectorPositionData"=FALSE, "TryMeasurementMode"=FALSE, "HasNivel"=FALSE, "HasVideoCamera"=FALSE} ("SystemSettingsData"), "ApplyTransformationParams"="Apply Transformation\nParameters") -> (w335:T20)
        n68 = call "SetSystemSettings.vi"("error in (no error)"=w339, "SystemSettingsData"=w335, "TCP Network Connection in"=w340) -> ("error out"=w337:errorcluster, "TCP Network Connection out"=w338:refnum<k5>)  [unwired: 5 in, 2 out]
      }
      frame "AddActualPoint" {
        n69 = local read "Actual Points"() -> (w350:T15)
        n70 = call "Eingabe Actual Point.vi"("error in (no error)"=w352, "TCP Network Connection in"=w355) -> ("error out"=w353:errorcluster, "Actual Point"=w351:T23, "TCP Network Connection out"=w354:refnum<k5>)  [unwired: 7 in]
        n71 = Build Array (concatenate)(w350, w351) -> (w349:T23[])
        n72 = Sort 1D Array(array=w349) -> (sorted array=w347:T23[])
        n73 = call "Schreibe Tabelle.vi"("Points"=w347) -> ("Table"=w348:T13)  [unwired: 10 in]
        n74 = local write "Actual Points Front Indicator"(w348) -> ()
        n75 = local write "Actual Points"(w347) -> ()
      }
      frame "CalcTransformation" {
        w379 = FALSE
        # "4."
        # "2."
        # "1. Aktuelle Transformation deaktivieren. Sonst wird Transformation auf Transformation\ngerechnet\n\n2. Löschen der bisherigen geladenen Soll- und Ist Koordinaten\n\n3. Laden der Soll- und Ist Koordinaten auf die Lasertracker Steuerung\n\n4. Berechnen der Transformationsparameter\n\n5. Setzen der Transformationsparameter"
        # "1."
        n76 = local read "Actual Points"() -> (w374:T15)
        n77 = local read "Nominal Points"() -> (w375:T15)
        n78 = local write "Apply Transformation\nParameters"(w379) -> ()
        n79 = Bundle By Name(cluster=T20 {"WeatherMonitorStatus"=enum."ES_WMS_ReadAndCalculateRefractions", "ApplyTransformationParams"=FALSE, "ApplyStationOrientationParams"=FALSE, "KeepLastPosition"=TRUE, "SendUnsolicitedMessages"=TRUE, "SendReflectorPositionData"=FALSE, "TryMeasurementMode"=FALSE, "HasNivel"=FALSE, "HasVideoCamera"=FALSE} ("SystemSettingsData"), "ApplyTransformationParams"=w379) -> (w386:T20)
        n80 = call "SortPoints.vi"("Nominal Points"=w375, "Actual Points"=w374) -> ("Nominal PointsOut"=w371:T15, "Actual Points Out"=w373:T15)  [unwired: 8 in]
        n81 = call "SetSystemSettings.vi"("error in (no error)"=w383, "SystemSettingsData"=w386, "TCP Network Connection in"=w382) -> ("error out"=w384:errorcluster, "TCP Network Connection out"=w385:refnum<k5>)  [unwired: 5 in, 2 out]
        n82 = Array Size(array=w373) -> (size(s)=w372:i32)
        n83 = call "ClearTransformationNominalPointList.vi"("error in (no error)"=w384, "TCP Network Connection in"=w385) -> ("error out"=w396:errorcluster, "TCP Network Connection out"=w397:refnum<k5>)  [unwired: 6 in, 2 out]
        n84 = call "ClearTransformationActualPointList.vi"("error in (no error)"=w396, "TCP Network Connection in"=w397) -> ("error out"=w394:errorcluster, "TCP Network Connection out"=w395:refnum<k5>)  [unwired: 6 in, 2 out]
        n85 = for {
          N: w372 -> [_]
          shift-right: [w403] -> w381
          shift-left: w395 -> [w407]
          shift-right: [w404] -> w380
          shift-left: w394 -> [w406]
          tunnel: w373 -> [w409] mode=indexing
          tunnel: w371 -> [w411] mode=indexing
          # "3."
          n86 = Unbundle By Name(w409) -> ("Transformation Point"=w408:T14)
          n87 = Unbundle By Name(w411) -> ("Transformation Point"=w410:T14)
          n88 = call "AddTransformationNominalPoint.vi"("error in (no error)"=w406, "Transformation Point"=w410, "TCP Network Connection in"=w407) -> ("error out"=w405:errorcluster, "TCP Network Connection out"=w402:refnum<k5>)  [unwired: 5 in, 2 out]
          n89 = call "AddTransformationActualPoint.vi"("error in (no error)"=w405, "Transformation Point"=w408, "TCP Network Connection in"=w402) -> ("error out"=w404:errorcluster, "TCP Network Connection out"=w403:refnum<k5>)  [unwired: 5 in, 2 out]
        }
        n90 = call "CallTransformation.vi"("error in (no error)"=w380, "TCP Network Connection in"=w381) -> ("error out"=w392:errorcluster, "CallTrafoCluster"=w389:T24, "TCP Network Connection out"=w393:refnum<k5>)  [unwired: 5 in, 2 out]
        n91 = Unbundle By Name(w389) -> ("dTransVal1"=w365:dbl, "dTransVal2"=w366:dbl, "dTransVal3"=w367:dbl, "dRot1"=w363:dbl, "dRot2"=w362:dbl, "dRot3"=w361:dbl, "dScale"=w368:dbl)
        "Scale" <- w368
        n92 = Build Array(w365, w366, w367) -> (→"Translation":dbl[])
        n93 = Bundle By Name(cluster=T22 {"dVal1"=2.0, "dVal2"=0.0, "dVal3"=5.0, "dRot1"=0.0, "dRot2"=0.0, "dRot3"=0.0, "dScale"=1.0} ("TransformationData"), "dVal1"=w365, "dVal2"=w366, "dVal3"=w367, "dRot1"=w363, "dRot2"=w362, "dRot3"=w361, "dScale"=w368) -> (w388:T22)
        n94 = call "SetTransformationParams.vi"("error in (no error)"=w392, "TransformationData"=w388, "TCP Network Connection in"=w393) -> ("error out"=w377:errorcluster, "TCP Network Connection out"=w391:refnum<k5>)  [unwired: 5 in, 2 out]
        n95 = Build Array(w363, w362, w361) -> (→"Rotation":dbl[])
        n96 = property on="CalcTransformation" class="Bool (strict)"(error in=w377, "Value"=FALSE ("CalcTransformation")) -> (error out=w376:errorcluster)  [unwired: 1 in, 1 out]
      }
      frame "PowerLock" {
        n97 = call "SetPowerLockFunctionActive.vi"("error in (no error)"=w417, "ES_BOOL"="SetPowerLock\nActive", "TCP Network Connection in"=w418) -> ("error out"=w414:errorcluster, "TCP Network Connection out"=w415:refnum<k5>)  [unwired: 5 in, 2 out]
      }
      frame "AddNominalPoint" {
        n98 = local read "Nominal Points"() -> (w428:T15)
        n99 = call "Eingabe Nominal Point.vi"() -> ("NominaPoint"=w429:T23)  [unwired: 11 in]
        n100 = Build Array (concatenate)(w428, w429) -> (w427:T23[])
        n101 = Sort 1D Array(array=w427) -> (sorted array=w426:T23[])
        n102 = call "Schreibe Tabelle.vi"("Points"=w426) -> ("Table"=w425:T13)  [unwired: 10 in]
        n103 = local write "Nominal Points"(w426) -> ()
        n104 = local write "Nominal Points Front Indicator"(w425) -> ()
      }
      frame "ClearLastActualPoint" {
        n105 = local read "Actual Points"() -> (w440:T15)
        n106 = Array Size(array=w440) -> (size(s)=w443:i32)
        n107 = Decrement(x=w443) -> (x-1=w442:i32)
        n108 = Array Subset(array=w440, index=0, length=w442) -> (w439:T15)
        n109 = local write "Actual Points"(w439) -> ()
        n110 = call "Schreibe Tabelle.vi"("Points"=w439) -> ("Table"=w438:T13)  [unwired: 10 in]
        n111 = local write "Actual Points Front Indicator"(w438) -> ()
      }
      frame "ClearLastNominalPoint" {
        n112 = local read "Nominal Points"() -> (w454:T15)
        n113 = Array Size(array=w454) -> (size(s)=w457:i32)
        n114 = Decrement(x=w457) -> (x-1=w456:i32)
        n115 = Array Subset(array=w454, index=0, length=w456) -> (w453:T15)
        n116 = local write "Nominal Points"(w453) -> ()
        n117 = call "Schreibe Tabelle.vi"("Points"=w453) -> ("Table"=w452:T13)  [unwired: 10 in]
        n118 = local write "Nominal Points Front Indicator"(w452) -> ()
      }
      frame "RemoveNominalByName" {
        n119 = local read "Nominal Points"() -> (w471:T15)
        n120 = call "RemoveByName.vi"("Nominal Points in"=w471, "Nominal to be Removes"="Nominal to be Removes") -> ("Nominal Points out"=w470:T15)  [unwired: 9 in]
        n121 = call "Schreibe Tabelle.vi"("Points"=w470) -> ("Table"=w472:T13)  [unwired: 10 in]
        n122 = local write "Nominal Points"(w470) -> ()
        n123 = local write "Nominal Points Front Indicator"(w472) -> ()
        n124 = property on="Remove Nominal by Name" class="Bool (strict)"(error in=w467, "Value"=FALSE ("Remove Nominal by Name")) -> (error out=w466:errorcluster)  [unwired: 1 in, 1 out]
      }
      frame "RemoveActualByName" {
        n125 = local read "Actual Points"() -> (w485:T15)
        n126 = call "RemoveByName.vi"("Nominal Points in"=w485, "Nominal to be Removes"="Actual to be Removed") -> ("Nominal Points out"=w483:T15)  [unwired: 9 in]
        n127 = call "Schreibe Tabelle.vi"("Points"=w483) -> ("Table"=w486:T13)  [unwired: 10 in]
        n128 = local write "Actual Points Front Indicator"(w486) -> ()
        n129 = local write "Actual Points"(w483) -> ()
        n130 = property on="Remove Actual by Name" class="Bool (strict)"(error in=w481, "Value"=FALSE ("Remove Actual by Name")) -> (error out=w482:errorcluster)  [unwired: 1 in, 1 out]
      }
      frame "AddNominalPointFile" {
        n131 = local read "Nominal Points"() -> (w498:T15)
        n132 = call "ReadPoints.vi"("Transform Points In"=w498) -> ("Transform Points out"=w497:T15)  [unwired: 10 in]
        n133 = Sort 1D Array(array=w497) -> (sorted array=w500:T15)
        n134 = call "Schreibe Tabelle.vi"("Points"=w500) -> ("Table"=w499:T13)  [unwired: 10 in]
        n135 = local write "Nominal Points Front Indicator"(w499) -> ()
        n136 = local write "Nominal Points"(w500) -> ()
        n137 = property on="Add Nominal File" class="Bool (strict)"(error in=w494, "Value"=FALSE ("Add Nominal File")) -> (error out=w493:errorcluster)  [unwired: 1 in, 1 out]
      }
      frame "AddActualPointFile" {
        n138 = local read "Actual Points"() -> (w507:T15)
        n139 = call "ReadPoints.vi"("Transform Points In"=w507) -> ("Transform Points out"=w513:T15)  [unwired: 10 in]
        n140 = Sort 1D Array(array=w513) -> (sorted array=w508:T15)
        n141 = call "Schreibe Tabelle.vi"("Points"=w508) -> ("Table"=w509:T13)  [unwired: 10 in]
        n142 = local write "Actual Points Front Indicator"(w509) -> ()
        n143 = local write "Actual Points"(w508) -> ()
        n144 = property on="Add Actual File" class="Bool (strict)"(error in=w511, "Value"=FALSE ("Add Actual File")) -> (error out=w510:errorcluster)  [unwired: 1 in, 1 out]
      }
      frame "ConnectTracker" {
        n145 = TCP Open Connection(address="IP Address", remote port or service name="Port", error in (no error)=w525) -> (connection ID=w526:refnum<k5>, error out=w523:errorcluster)  [unwired: 2 in]
        n146 = property on="Connect" class="Bool (strict)"(error in=w523, "Value"=FALSE ("Connect")) -> (error out=w522:errorcluster)  [unwired: 1 in, 1 out]
      }
      frame "PlotValueChange" {
        n147 = Index Array(array=w544, index (col) #1=0 ("disabled index (col)"), index (col) #2=1 ("index (col)")) -> (element #1=w542:dbl[], element #2=w541:dbl[])  [unwired: 2 in]
        n148 = call-poly <vilib>:"Mean.vi"("X"=w542) -> ("mean"=w535:dbl)  [unwired: 1 out]
        n149 = call-poly <vilib>:"Mean.vi"("X"=w541) -> ("mean"=w538:dbl)  [unwired: 1 out]
        n150 = Subtract(x=w538, y="Axis Scaling") -> (x-y=w537:dbl)
        n151 = Subtract(x=w535, y="Axis Scaling") -> (x-y=w539:dbl)
        n152 = Add(x=w538, y="Axis Scaling") -> (x+y=w536:dbl)
        n153 = Add(x=w535, y="Axis Scaling") -> (x+y=w540:dbl)
        n154 = property on="XY Graph" class="XYGraph (strict)"(error in=w547, "XScale.Maximum"=w540, "XScale.Minimum"=w539, "YScale.Maximum"=w536, "YScale.Minimum"=w537) -> (error out=w546:errorcluster)  [unwired: 1 in, 1 out]
      }
    }
    n155 = call "PlotPoints.vi"("Array"=w38) -> ("XY Graph"=→"XY Graph":cluster{"Array":dbl[], "Array 3":dbl[]})  [unwired: 10 in]
  }
  n156 = while {
    tunnel: w30 -> [w563]
    tunnel: w29 -> [w562]
    tunnel: [w561] -> w32
    tunnel: [w560] -> w31
    stop <- w559 stop-if-true
    # "Schleife zur Erfassung von Eingaben (Producer)"
    n157 = event shown="[12] \"Add Actual File\": Mouse Down" {
      selector: _ -> [_ _ _ _ _ _ _ _ _ _ _ _ _ _ _ _ _ _ _ _ _ _ _ _ _]
      dyn-events: _ -> [_ _ _ _ _ _ _ _ _ _ _ _ _ _ _ _ _ _ _ _ _ _ _ _ _]
      timeout: _ -> [_ _ _ _ _ _ _ _ _ _ _ _ _ _ _ _ _ _ _ _ _ _ _ _ _]
      tunnel: w563 -> [w565 w567 w573 w578 w583 w586 w593 w602 w607 w614 w621 w623 w631 w636 w641 w646 w651 w659 w663 w669 w672 w679 w684 w689 w694]
      tunnel: w562 -> [w564 w566 w572 w577 w582 w588 w592 w601 w608 w612 w620 w624 w630 w635 w640 w645 w652 w658 w662 w668 w671 w678 w683 w686 w693]
      tunnel: [w565 w567 w571 w576 w580 w585 w594 w600 w609 w610 w619 w626 w629 w634 w639 w644 w654 w657 w660 w667 w673 w676 w682 w688 w692] -> w561
      tunnel: [w564 w566 w570 w575 w579 w590 w597 w603 w605 w611 w616 w625 w628 w633 w638 w643 w653 w656 w661 w666 w674 w677 w681 w687 w691] -> w560
      tunnel: [_ TRUE _ _ _ _ _ _ _ _ _ _ _ _ _ _ _ _ _ _ _ _ _ _ _] -> w559
      event Timeout {
        n158 = event-data() -> ()  [unwired: 1 in, 3 out]
      }
      event Panel Close {
        n159 = event-data() -> ()  [unwired: 1 in, 4 out]
      }
      event "Connect": Mouse Down {
        n160 = event-data() -> ()  [unwired: 1 in, 7 out]
        n161 = Enqueue Element(queue=w573, element=Queue_Steuerung_Commands."ConnectTracker", error in (no error)=w572) -> (queue out=w571:refnum<queue>, error out=w570:errorcluster)  [unwired: 1 in, 1 out]
      }
      event "Initialize": Mouse Down {
        n162 = event-data() -> ()  [unwired: 1 in, 2 out]
        n163 = Enqueue Element(queue=w578, element=Queue_Steuerung_Commands."Initialise", error in (no error)=w577) -> (queue out=w576:refnum<queue>, error out=w575:errorcluster)  [unwired: 1 in, 1 out]
      }
      event "Apply Transformation\nParameters": Value Change {
        n164 = event-data() -> ()  [unwired: 1 in, 3 out]
        n165 = Enqueue Element(queue=w583, element=Queue_Steuerung_Commands."Punkte Transformieren", error in (no error)=w582) -> (queue out=w580:refnum<queue>, error out=w579:errorcluster)  [unwired: 1 in, 1 out]
      }
      event "Add Nominal": Mouse Down {
        n166 = event-data() -> ()  [unwired: 1 in, 3 out]
        n167 = Enqueue Element(queue=w586, element=Queue_Steuerung_Commands."AddNominalPoint", error in (no error)=w588) -> (queue out=w585:refnum<queue>, error out=w587:errorcluster)  [unwired: 1 in, 1 out]
        n168 = property on="Add Nominal" class="Bool (strict)"(error in=w587, "Value"=FALSE ("Add Nominal")) -> (error out=w590:errorcluster)  [unwired: 1 in, 1 out]
      }
      event "Clear Nominal": Mouse Down {
        n169 = event-data() -> ()  [unwired: 1 in, 3 out]
        n170 = Enqueue Element(queue=w593, element=Queue_Steuerung_Commands."ClearLastNominalPoint", error in (no error)=w592) -> (queue out=w594:refnum<queue>, error out=w595:errorcluster)  [unwired: 1 in, 1 out]
        n171 = property on="Clear Nominal" class="Bool (strict)"(error in=w595, "Value"=FALSE ("Clear Nominal")) -> (error out=w597:errorcluster)  [unwired: 1 in, 1 out]
      }
      event "Clear Actual": Mouse Down {
        n172 = event-data() -> ()  [unwired: 1 in, 7 out]
        n173 = Enqueue Element(queue=w602, element=Queue_Steuerung_Commands."ClearLastActualPoint", error in (no error)=w601) -> (queue out=w600:refnum<queue>, error out=w599:errorcluster)  [unwired: 1 in, 1 out]
        n174 = property on="Clear Actual" class="Bool (strict)"(error in=w599, "Value"=FALSE ("Clear Actual")) -> (error out=w603:errorcluster)  [unwired: 1 in, 1 out]
      }
      event "CalcTransformation": Mouse Down {
        n175 = event-data() -> ()  [unwired: 1 in, 7 out]
        n176 = Enqueue Element(queue=w607, element=Queue_Steuerung_Commands."CalcTransformation", error in (no error)=w608) -> (queue out=w609:refnum<queue>, error out=w605:errorcluster)  [unwired: 1 in, 1 out]
      }
      event "GoBirdBath": Mouse Down {
        n177 = event-data() -> ()  [unwired: 1 in, 2 out]
        n178 = Enqueue Element(queue=w614, element=Queue_Steuerung_Commands."GoBirdBath", error in (no error)=w612) -> (queue out=w610:refnum<queue>, error out=w611:errorcluster)  [unwired: 1 in, 1 out]
      }
      event "Add Actual Point": Mouse Down {
        n179 = event-data() -> ()  [unwired: 1 in, 7 out]
        n180 = Enqueue Element(queue=w621, element=Queue_Steuerung_Commands."AddActualPoint", error in (no error)=w620) -> (queue out=w619:refnum<queue>, error out=w617:errorcluster)  [unwired: 1 in, 1 out]
        n181 = property on="Add Actual Point" class="Bool (strict)"(error in=w617, "Value"=FALSE ("Add Actual Point")) -> (error out=w616:errorcluster)  [unwired: 1 in, 1 out]
      }
      event "SingleMeas": Mouse Down {
        n182 = event-data() -> ()  [unwired: 1 in, 2 out]
        n183 = Enqueue Element(queue=w623, element=Queue_Steuerung_Commands."SingleMeasurement", error in (no error)=w624) -> (queue out=w626:refnum<queue>, error out=w625:errorcluster)  [unwired: 1 in, 1 out]
      }
      event "Add Actual File": Mouse Down {
        n184 = event-data() -> ()  [unwired: 1 in, 7 out]
        n185 = Enqueue Element(queue=w631, element=Queue_Steuerung_Commands."AddActualPointFile", error in (no error)=w630) -> (queue out=w629:refnum<queue>, error out=w628:errorcluster)  [unwired: 1 in, 1 out]
      }
      event "Remove Nominal by Name": Mouse Down {
        n186 = event-data() -> ()  [unwired: 1 in, 7 out]
        n187 = Enqueue Element(queue=w636, element=Queue_Steuerung_Commands."RemoveNominalByName", error in (no error)=w635) -> (queue out=w634:refnum<queue>, error out=w633:errorcluster)  [unwired: 1 in, 1 out]
      }
      event "Remove Actual by Name": Mouse Down {
        n188 = event-data() -> ()  [unwired: 1 in, 7 out]
        n189 = Enqueue Element(queue=w641, element=Queue_Steuerung_Commands."RemoveActualByName", error in (no error)=w640) -> (queue out=w639:refnum<queue>, error out=w638:errorcluster)  [unwired: 1 in, 1 out]
      }
      event "Add Nominal File": Mouse Down {
        n190 = event-data() -> ()  [unwired: 1 in, 7 out]
        n191 = Enqueue Element(queue=w646, element=Queue_Steuerung_Commands."AddNominalPointFile", error in (no error)=w645) -> (queue out=w644:refnum<queue>, error out=w643:errorcluster)  [unwired: 1 in, 1 out]
      }
      event "ContMeas": Mouse Down {
        n192 = event-data() -> ()  [unwired: 1 in, 2 out]
        n193 = Select(t=Queue_Steuerung_Commands."StopContMeas", s="ContMeas", f=Queue_Steuerung_Commands."StartContMeas") -> (s? t:f=w649:T16)
        n194 = Enqueue Element(queue=w651, element=w649, error in (no error)=w652) -> (queue out=w654:refnum<queue>, error out=w653:errorcluster)  [unwired: 1 in, 1 out]
      }
      event Value Change {
        n195 = event-data() -> ()  [unwired: 1 in, 2 out]
        n196 = Enqueue Element(queue=w659, element=Queue_Steuerung_Commands."SetUnits", error in (no error)=w658) -> (queue out=w657:refnum<queue>, error out=w656:errorcluster)  [unwired: 1 in, 1 out]
      }
      event Value Change {
        n197 = event-data() -> ()  [unwired: 1 in, 2 out]
        n198 = Enqueue Element(queue=w663, element=Queue_Steuerung_Commands."SetCoordType", error in (no error)=w662) -> (queue out=w660:refnum<queue>, error out=w661:errorcluster)  [unwired: 1 in, 1 out]
      }
      event "GetEnvParams": Mouse Down {
        n199 = event-data() -> ()  [unwired: 1 in, 2 out]
        n200 = Enqueue Element(queue=w669, element=Queue_Steuerung_Commands."GetEnvParams", error in (no error)=w668) -> (queue out=w667:refnum<queue>, error out=w666:errorcluster)  [unwired: 1 in, 1 out]
      }
      event "Axis Scaling": Value Change {
        n201 = event-data() -> ()  [unwired: 1 in, 6 out]
        n202 = Enqueue Element(queue=w672, element=Queue_Steuerung_Commands."PlotValueChange", error in (no error)=w671) -> (queue out=w673:refnum<queue>, error out=w674:errorcluster)  [unwired: 1 in, 1 out]
      }
      event Value Change {
        n203 = event-data() -> ()  [unwired: 1 in, 2 out]
        n204 = Enqueue Element(queue=w679, element=Queue_Steuerung_Commands."SetStatMeasParams", error in (no error)=w678) -> (queue out=w676:refnum<queue>, error out=w677:errorcluster)  [unwired: 1 in, 1 out]
      }
      event Value Change {
        n205 = event-data() -> ()  [unwired: 1 in, 2 out]
        n206 = Enqueue Element(queue=w684, element=Queue_Steuerung_Commands."SetReflector", error in (no error)=w683) -> (queue out=w682:refnum<queue>, error out=w681:errorcluster)  [unwired: 1 in, 1 out]
      }
      event "Continuous Time Mode Params": Value Change {
        n207 = event-data() -> ()  [unwired: 1 in, 6 out]
        n208 = Enqueue Element(queue=w689, element=Queue_Steuerung_Commands."SetContTimeParams", error in (no error)=w686) -> (queue out=w688:refnum<queue>, error out=w687:errorcluster)  [unwired: 1 in, 1 out]
      }
      event "SetPowerLock\nActive": Value Change {
        n209 = event-data() -> ()  [unwired: 1 in, 6 out]
        n210 = Enqueue Element(queue=w694, element=Queue_Steuerung_Commands."PowerLock", error in (no error)=w693) -> (queue out=w692:refnum<queue>, error out=w691:errorcluster)  [unwired: 1 in, 1 out]
      }
    }
  }
  n211 = Release Queue(queue=w32, error in (no error)=w31) -> (error out=w19:errorcluster)  [unwired: 1 in, 2 out]
  n212 = call "StopMeasurement.vi"("error in (no error)"=w11, "TCP Network Connection in"=w8) -> ("error out"=w10:errorcluster, "TCP Network Connection out"=w9:refnum<k5>)  [unwired: 6 in, 2 out]
  n213 = Release Queue(queue=w23, error in (no error)=w22) -> (error out=w21:errorcluster)  [unwired: 1 in, 2 out]
  n214 = TCP Close Connection(connection ID=w9, error in (no error)=w10) -> (error out=w20:errorcluster)  [unwired: 1 in, 1 out]
  n215 = Close File(refnum=w17, error in=w1) -> (error out=w15:errorcluster)  [unwired: 1 out]
  n216 = Merge Errors(w19, w20, w21, w15) -> (w12:errorcluster)
  n217 = call <vilib>:"Simple Error Handler.vi"("error in (no error)"=w12) -> ()  [unwired: 4 in, 5 out]
  "Actual Points" <- w14
  "Nominal Points" <- w14
  "Nominal Points Front Indicator" <- w13
  "Actual Points Front Indicator" <- w13
